vi "ME_acquire_13_DeltaForce_Daq.vi"() -> ()   [LabVIEW 2015]
doc: "Use this template to build a producer/consumer design pattern. Use this template when you need to execute a process, such as data analysis, when a data source, such as a triggered acquisition, produces data at an uneven rate and you need to execute the process when the data becomes available."
uses:
  Mode.ctl
  oxford_driver/Oxford Drivers/BUSGEN.LLB/OxfordAddress.ctl
  <vilib>/Analysis/baseanly.llb/Mean (DBL).vi
  <vilib>/DAQmx/read.llb/DAQmx Read (Analog 1D DBL 1Chan NSamp).vi
  <vilib>/DAQmx/create/channels.llb/DAQmx Create Channel (AI-Voltage-Basic).vi
  <vilib>/DAQmx/configure/timing.llb/DAQmx Timing (Sample Clock).vi
  <vilib>/Utility/file.llb/Write Delimited Spreadsheet (DBL).vi
  <vilib>/DAQmx/miscellaneous.llb/DAQmx Fill In Error Info.vi
  <vilib>/express/express arith-compare/Formula/XNode/ExpressFormulaBlockNode.xnode
  <vilib>/Analysis/NI_AALBase.lvlib
panel:
  out "concatenated string":string
  out "remaining elements 2":T1(array[cluster])
  out "Actual mean":dbl format="%0.6f"
  in  "Averaged dt":dbl[][](array[numeric])
  in  "Averaged P(B)":dbl[][](array[numeric])
  out "LockInR":dbl
  out "deltaUaux":dbl
  out "Actual Voltage (V)":dbl caption="Actual AuxV" step=0.1
  in  "Stop":bool
  out "SaveSweep":bool=TRUE
  out "Measurement File_dn":path
  out "Measurement File_up":path
  out "Measurement File_average":path
  out "Actual Polarization":dbl
  in  "Reset IB?":bool
  in  "First?":bool
  in  "Save Period":dbl=1.0
  out "Averaged I(B)":dbl[][](array[numeric])
  out "P(uC/mm^2)":dbl[](array[numeric])
  in  "Sweep":bool
  out "Offset array":dbl[](array[numeric])
  in  "stop 2":bool
  in  "dB":dbl=0.005
  out "appended array":dbl[][](array[numeric])
  out "Actual B Field (T)":dbl
  out "Actual Temperature (K)":dbl
  out "Actual Current (pA)":dbl
  in  "Tab Control":T2(tab)
  in  "Max temperature (K)":dbl=20.0
  in  "Min Temperature (K)":dbl=4.5
  out "P(T)":cluster{"yi":dbl[], dbl[]}(graph)
  out "I(T)":cluster{dbl[], dbl[]}(graph)
  in  "Set temperature (K)":dbl=4.5
  in  "Temp Ramping Rate (K/min)":dbl=10.0
  in  "Heater Range":enum16{"Off", "Low", "Medium", "High"}(ring)
  in  "Heater On/Off":bool
  out "Setpoint Temperature (K)":dbl
  out "I(B) 3":cluster{dbl[], dbl[]}[](graph)
  out "I(B) /Averaged/":cluster{"B array":dbl[], dbl[]}[](graph)
  out "P(B) /Averaged/":cluster{"B array":dbl[], dbl[]}[](graph)
  out "P(B)":cluster{"yi":dbl[], dbl[]}(graph)
  in  "Set Field (T)":dbl
  in  "Go to Set":bool
  in  "Sweep Rate (T/min)":dbl=2.0 format="%.6f"
  in  "Field To Zero":bool
  out "Target Field":dbl
  in  "Min Field (T)":dbl
  in  "Max Field (T)":dbl=0.15
  in  "Threshold B (T)":dbl
  out "Up/Down":bool
  in  "Max count array":i32[](array[numeric])=[2, 1, 0, 0, 0, 9, 10, 11, 12]
  in  "secs to wait":dbl=180.0
  out "Wait (s)":dbl
  in  "Directory":string
  out "Finished":bool=TRUE
  out "Step Rate":bool
  out "New":bool=TRUE
  in  "Temperature Array":dbl[](array[numeric])=[4.5, 5.0, 6.0, 7.0, 8.0, 9.0, 10.0, 11.0, 12.0]
  in  "Sweep Rate Array":dbl[](array[numeric])=[2.0, 1.0, 0.5, 0.1, 0.05, 9.0, 10.0, 11.0, 12.0]
  in  "Record ALL":bool
  in  "Max Countl":i32
  out "i":i32
  out "j":i32
  out "Step Temp":bool
  in  "FileName":string
  in  "Measure Noise":bool
  in  "Cycles":i32
  in  "maximum value":dbl=10.0 format="%0.2f"
  in  "minimum value":dbl=-10.0 format="%0.2f"
  in  "physical channels":tag="Dev1/ai1"
  out "PSD (pA/Hz^1/2) Peaks Removed":cluster{"f0":dbl, "df":dbl, "magnitude":dbl[]}(graph)
  out "PSD (pA/Hz^1/2)":cluster{"f0":dbl, "df":dbl, "magnitude":dbl[]}(graph)
  out "Current (pA) Filtered":waveform(dbl)(graph)
  out "Current (pA)":dbl[](graph)
  in  "Samples per channel":i32=1000
  in  "Rate":dbl=1000.0 format="%0.2f"
  in  "Cut-Off Frequency":dbl=100.0 caption="Lower Cut-Off"
  in  "Filter On":bool
  in  "Keithley (IV conv) averaging":i32=10
  in  "Lock_in_Amplifier":refnum<visa-resource-name>="GPIB0::5::INSTR"
  out "Dc offset":dbl
  in  "Calibrate":bool
  in  "IV converter":refnum<visa-resource-name>="GPIB0::20::INSTR"
  in  "Magnetic Field":refnum<visa-resource-name>="GPIB0::21::INSTR"
  out "Time Lag":dbl=0.0500025749206543
  in  "Lake Shore":refnum<visa-resource-name>="GPIB0::11::INSTR"
  in  "Temp Refresh (s)":dbl=0.1
  in  "Sampling rate (Hz)":dbl=10.0
  in  "Gain (V/A)":dbl=1000000000.0
  in  "Sample area (mm^2)":dbl=1.0
  out "B_V":cluster{dbl[], "Best Linear Fit":dbl[]}[](graph)=[{[-0.00769241141, -0.00768011662, -0.0029394633, 0.00271952438, 0.00937200583, 0.0154641889, 0.0217080684, 0.0281692221, 0.0344763397, 0.0407091529, 0.0473661569, 0.0541476438, 0.0611164384, 0.0676637725, 0.073937413, 0.0801511723, 0.0863882257, 0.0933787866, 0.0997676928, 0.106163316, 0.113953626, 0.118979018, 0.126030157, 0.132855724, 0.13883398, 0.14631074, 0.153030676, 0.159156864, 0.165801088, 0.17248087, 0.178555009, 0.185285367, 0.192834407, 0.198751051, 0.205413053, 0.212847389, 0.219477697, 0.225574642, 0.232225854, 0.239015189, 0.245675966, 0.252411162, 0.258453848, 0.265211852, 0.271251534, 0.277801221, 0.284008329, 0.291402813, 0.297970768, 0.304082546, 0.310761405, 0.317366634, 0.323522001, 0.330123184, 0.336841279, 0.343557963, 0.349608435, 0.356238003, 0.363590921, 0.370338319, 0.376962983], "Best Linear Fit"=[0.0, 0.0015, 0.0035, 0.0056, 0.0076, 0.0096, 0.0116, 0.0136, 0.0156, 0.0177, 0.0197, 0.0219, 0.0239, 0.0259, 0.0279, 0.0299, 0.032, 0.034, 0.036, 0.038, 0.04, 0.042, 0.0441, 0.046, 0.048, 0.05, 0.052, 0.054, 0.056, 0.058, 0.06, 0.0621, 0.0643, 0.0663, 0.0684, 0.0704, 0.0725, 0.0745, 0.0765, 0.0787, 0.0807, 0.0827, 0.0847, 0.0868, 0.0888, 0.0908, 0.0928, 0.0948, 0.0968, 0.0988, 0.1008, 0.1028, 0.1048, 0.1069, 0.1091, 0.1111, 0.1131, 0.1152, 0.1173, 0.1193, 0.1213]}, {[-0.00769241141, -0.00768011662, -0.0029394633, 0.00271952438, 0.00937200583, 0.0154641889, 0.0217080684, 0.0281692221, 0.0344763397, 0.0407091529, 0.0473661569, 0.0541476438, 0.0611164384, 0.0676637725, 0.073937413, 0.0801511723, 0.0863882257, 0.0933787866, 0.0997676928, 0.106163316, 0.113953626, 0.118979018, 0.126030157, 0.132855724, 0.13883398, 0.14631074, 0.153030676, 0.159156864, 0.165801088, 0.17248087, 0.178555009, 0.185285367, 0.192834407, 0.198751051, 0.205413053, 0.212847389, 0.219477697, 0.225574642, 0.232225854, 0.239015189, 0.245675966, 0.252411162, 0.258453848, 0.265211852, 0.271251534, 0.277801221, 0.284008329, 0.291402813, 0.297970768, 0.304082546, 0.310761405, 0.317366634, 0.323522001, 0.330123184, 0.336841279, 0.343557963, 0.349608435, 0.356238003, 0.363590921, 0.370338319, 0.376962983], "Best Linear Fit"=[0.002353460844818253, 0.002357267374965663, 0.003824997997530172, 0.005577049655813272, 0.007636692089275871, 0.009522863265806463, 0.01145600043639222, 0.013456406815525209, 0.015409122826751182, 0.01733883381400479, 0.019399876452181594, 0.021499459635718428, 0.023657034245452215, 0.025684122519169482, 0.027626473848249778, 0.02955028565017564, 0.03148130942513291, 0.03364562299316916, 0.03562366117513693, 0.037603778974812686, 0.040015698972850115, 0.04157158615356273, 0.04375465501257369, 0.04586788562152819, 0.0477187843918964, 0.050033627699098075, 0.05211415440778254, 0.05401085368533849, 0.056067939569859164, 0.05813603439385595, 0.06001661903361471, 0.06210037244704129, 0.06443759401357516, 0.0662694173922171, 0.06833200743687069, 0.07063371605572277, 0.07268649347515121, 0.0745741389696738, 0.07663338837489471, 0.07873540137051047, 0.08079761214887074, 0.08288286343195213, 0.08475371006132383, 0.08684602281837933, 0.08871593939391825, 0.09074375613756333, 0.09266550866283872, 0.09495487889775463, 0.09698835150804998, 0.09888058937557581, 0.10094839843403076, 0.10299341126621803, 0.10489914451207855, 0.10694290468187984, 0.10902286140750632, 0.11110238128028392, 0.11297563849525552, 0.11502818680688229, 0.1173046879946565, 0.11939371707962458, 0.12144474708765744]}]
  out "V_I":cluster{dbl[], "Best Linear Fit":dbl[]}[](graph)=[{[0.0, 0.012, 0.026, 0.04, 0.054, 0.068, 0.081, 0.096, 0.11, 0.124, 0.138, 0.153, 0.167, 0.18, 0.195, 0.208, 0.223, 0.236, 0.251, 0.265, 0.279, 0.292, 0.306, 0.32, 0.334, 0.348, 0.362, 0.375, 0.389, 0.403, 0.417, 0.432, 0.446, 0.46, 0.475, 0.489, 0.504, 0.517, 0.531, 0.546, 0.56, 0.574, 0.588, 0.602, 0.616, 0.63, 0.644, 0.658, 0.672, 0.685, 0.699, 0.713, 0.727, 0.742, 0.755, 0.77, 0.784, 0.799, 0.814, 0.827, 0.841], "Best Linear Fit"=[-0.00769241141, -0.00768011662, -0.0029394633, 0.00271952438, 0.00937200583, 0.0154641889, 0.0217080684, 0.0281692221, 0.0344763397, 0.0407091529, 0.0473661569, 0.0541476438, 0.0611164384, 0.0676637725, 0.073937413, 0.0801511723, 0.0863882257, 0.0933787866, 0.0997676928, 0.106163316, 0.113953626, 0.118979018, 0.126030157, 0.132855724, 0.13883398, 0.14631074, 0.153030676, 0.159156864, 0.165801088, 0.17248087, 0.178555009, 0.185285367, 0.192834407, 0.198751051, 0.205413053, 0.212847389, 0.219477697, 0.225574642, 0.232225854, 0.239015189, 0.245675966, 0.252411162, 0.258453848, 0.265211852, 0.271251534, 0.277801221, 0.284008329, 0.291402813, 0.297970768, 0.304082546, 0.310761405, 0.317366634, 0.323522001, 0.330123184, 0.336841279, 0.343557963, 0.349608435, 0.356238003, 0.363590921, 0.370338319, 0.376962983]}, {[0.0, 0.012, 0.026, 0.04, 0.054, 0.068, 0.081, 0.096, 0.11, 0.124, 0.138, 0.153, 0.167, 0.18, 0.195, 0.208, 0.223, 0.236, 0.251, 0.265, 0.279, 0.292, 0.306, 0.32, 0.334, 0.348, 0.362, 0.375, 0.389, 0.403, 0.417, 0.432, 0.446, 0.46, 0.475, 0.489, 0.504, 0.517, 0.531, 0.546, 0.56, 0.574, 0.588, 0.602, 0.616, 0.63, 0.644, 0.658, 0.672, 0.685, 0.699, 0.713, 0.727, 0.742, 0.755, 0.77, 0.784, 0.799, 0.814, 0.827, 0.841], "Best Linear Fit"=[-0.015941127780698654, -0.010342478990544012, -0.0038107220686969304, 0.0027210348531501527, 0.009252791774997235, 0.01578454869684432, 0.02184975155284518, 0.028848062540538483, 0.03537981946238557, 0.041911576384232645, 0.048443333306079736, 0.05544164429377303, 0.061973401215620116, 0.06803860407162098, 0.07503691505931429, 0.08110211791531513, 0.08810042890300844, 0.0941656317590093, 0.10116394274670261, 0.1076956996685497, 0.11422745659039678, 0.12029265944639762, 0.1268244163682447, 0.1333561732900918, 0.13988793021193888, 0.14641968713378595, 0.15295144405563305, 0.15901664691163392, 0.165548403833481, 0.1720801607553281, 0.17861191767717516, 0.18561022866486845, 0.19214198558671555, 0.19867374250856262, 0.20567205349625592, 0.212203810418103, 0.2192021214057963, 0.22526732426179719, 0.23179908118364426, 0.23879739217133758, 0.24532914909318465, 0.2518609060150317, 0.2583926629368788, 0.2649244198587259, 0.271456176780573, 0.27798793370242003, 0.28451969062426713, 0.29105144754611423, 0.2975832044679613, 0.3036484073239622, 0.31018016424580924, 0.3167119211676563, 0.3232436780895034, 0.3302419890771967, 0.3363071919331976, 0.3433055029208909, 0.34983725984273795, 0.35683557083043127, 0.36383388181812454, 0.3698990846741254, 0.3764308415959725]}]
  out "B0 (T)":dbl=0.0026443907573365636
  out "B/V (T/V)":dbl=0.3027997253900218
  out "I0 (A)":dbl=-0.008736391445912099
  out "V/I (Ohm)":dbl=0.4773805959957447
  in  "Offset?":bool
  in  "Magnet":bool=TRUE
  in  "Ramp":bool=TRUE
  in  "DaQ":bool
  in  "Moving average":i8=10
  in  "Sample Rate":dbl=1000.0
  in  "Number of Samples":i32=100
  in  "Physical Channel":tag="kartya/ai0"
  in  "Min Voltage":dbl=-5.0
  in  "Max Voltage":dbl=5.0
  in  "Terminal Configuration":i32(ring)=-1 items=["default"=-1, "RSE"=10083, "NRSE"=10078, "Differential"=10106, "Pseudodifferential"=12529]
  out "Confirm":bool
  in  "Dwell Time (ms)":u32=1000
  in  "Temp/Magnetic Field":bool
  out "index":i8
  out "Read?":bool
  out "Magnetic Field (T)":dbl[](array[numeric])
  out "Reset":bool
  out "Measured Current (pA)":dbl[](array[numeric])
  out "Elapsed Time (s)":dbl[](array[numeric])
  out "Start time":timestamp
  in  "Enum":T3=enum."Process"
  out "B array":dbl[](array[numeric])
  in  "dB (T)":dbl=0.0025
  in  "Counter":i8
  out "L magnet (H)":dbl
  out "R magnet (mOhm)":dbl
  out "Actual Current (R0)":dbl
  out "Actual Field (T)":dbl
  out "Temperature array":dbl[](array[numeric])
  in  "New Measurement File":bool
  out "Measurement File":path
  out "refnum out":refnum<file>
  in  "Measuring":bool
  in  "Measure /Pause":bool
  in  "stop":bool
  # "DeltaForce"
  # "Discrete"
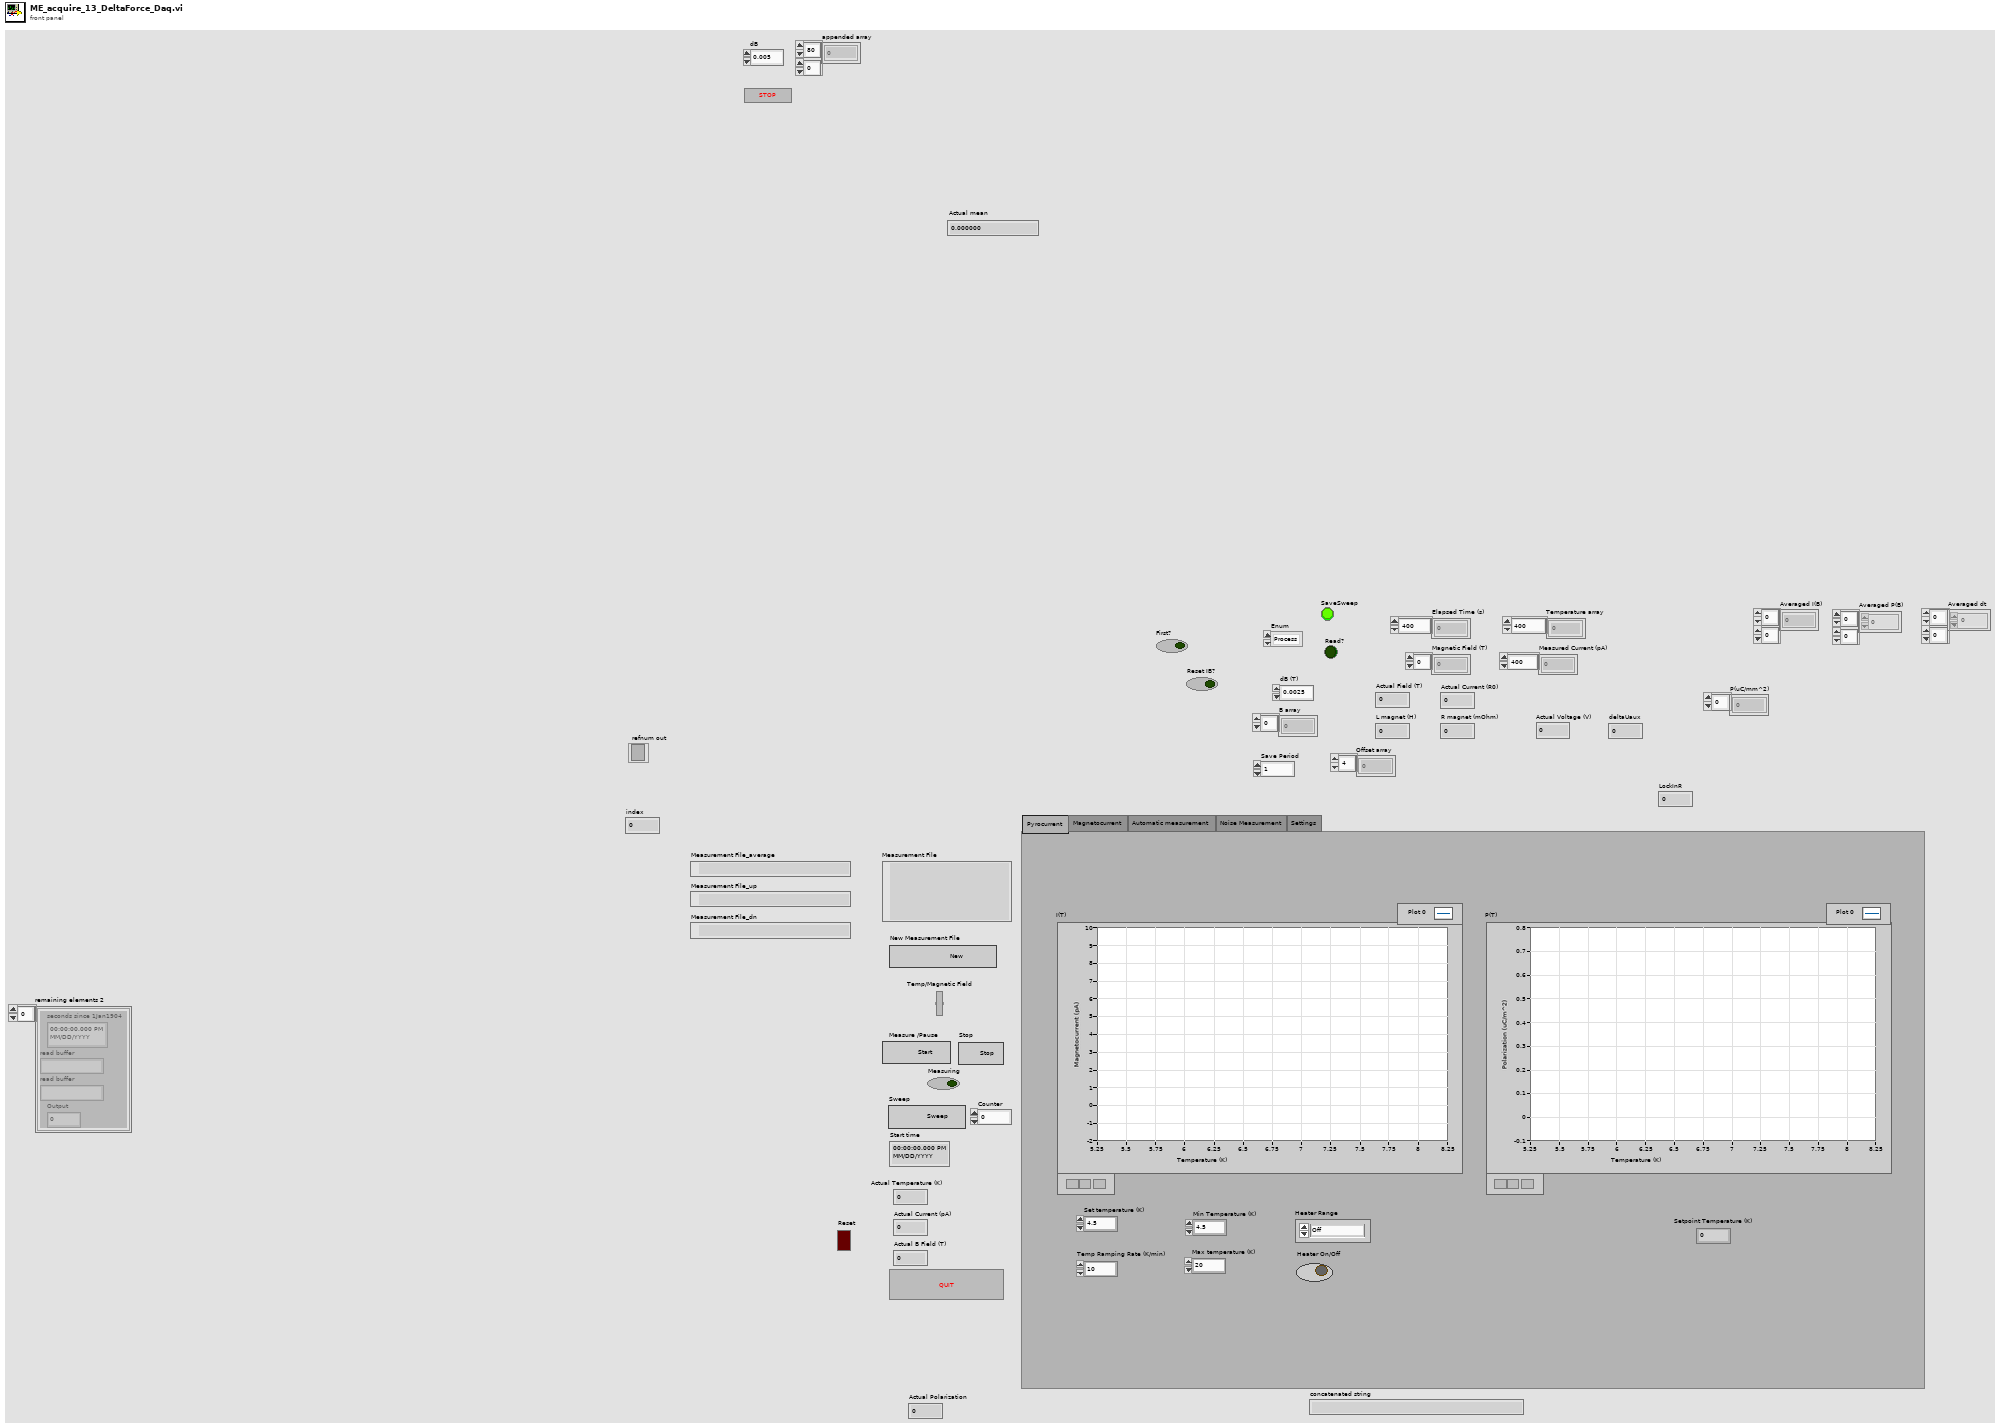
[diagram p1: front panel]
types:
  T1 = cluster{"seconds since 1Jan1904":timestamp, "read buffer":string, "read buffer":string, "Output":dbl}[]
  T2 = enum32{"Pyrocurrent", "Magnetocurrent", "Automatic measurement", "Noise Measurement", "Settings"}
  T3 = typedef "Mode.ctl" = enum16{"Offset", "Process", "Sweep", "StepOxford", "StepDelta", "Plot", "Save", "New", "Return", ""}
  T4 = cluster{"seconds since 1Jan1904":timestamp, "read buffer":string, "read buffer":string, "Output":dbl}
  T5 = enum16{"open", "replace", "create", "open or create", "replace or create", "replace or create with confirmation"}
  T6 = typedef "OxfordAddress.ctl" = cluster{"Com Port":i32, "ISOBUS Address":i32, "GPIB Address":i16, "Communication":enum16{"RS232", "ISOBUS", "GPIB", "Gateway"}}
  T7 = cluster{"B array":dbl[], "Averaged P(B) Out":dbl[]}
  T8 = cluster{"B array":dbl[], "BaselineSubtracted I(B)":dbl[]}
  T9 = cluster{"B array":dbl[], "Averaged P(B) Out":dbl[]}[]
  T10 = cluster{"B array":dbl[], "BaselineSubtracted I(B)":dbl[]}[]
  T11 = cluster{"I array out (A)":dbl[], "V array out (V)":dbl[]}
  T12 = cluster{"I array out (A)":dbl[], "Best Linear Fit":dbl[]}
  T13 = cluster{"V array out (V)":dbl[], "B array Out":dbl[]}
  T14 = cluster{"V array out (V)":dbl[], "Best Linear Fit 2":dbl[]}
  T15 = cluster{"I array out (A)":dbl[], "Best Linear Fit":dbl[]}[]
  T16 = cluster{"V array out (V)":dbl[], "Best Linear Fit 2":dbl[]}[]
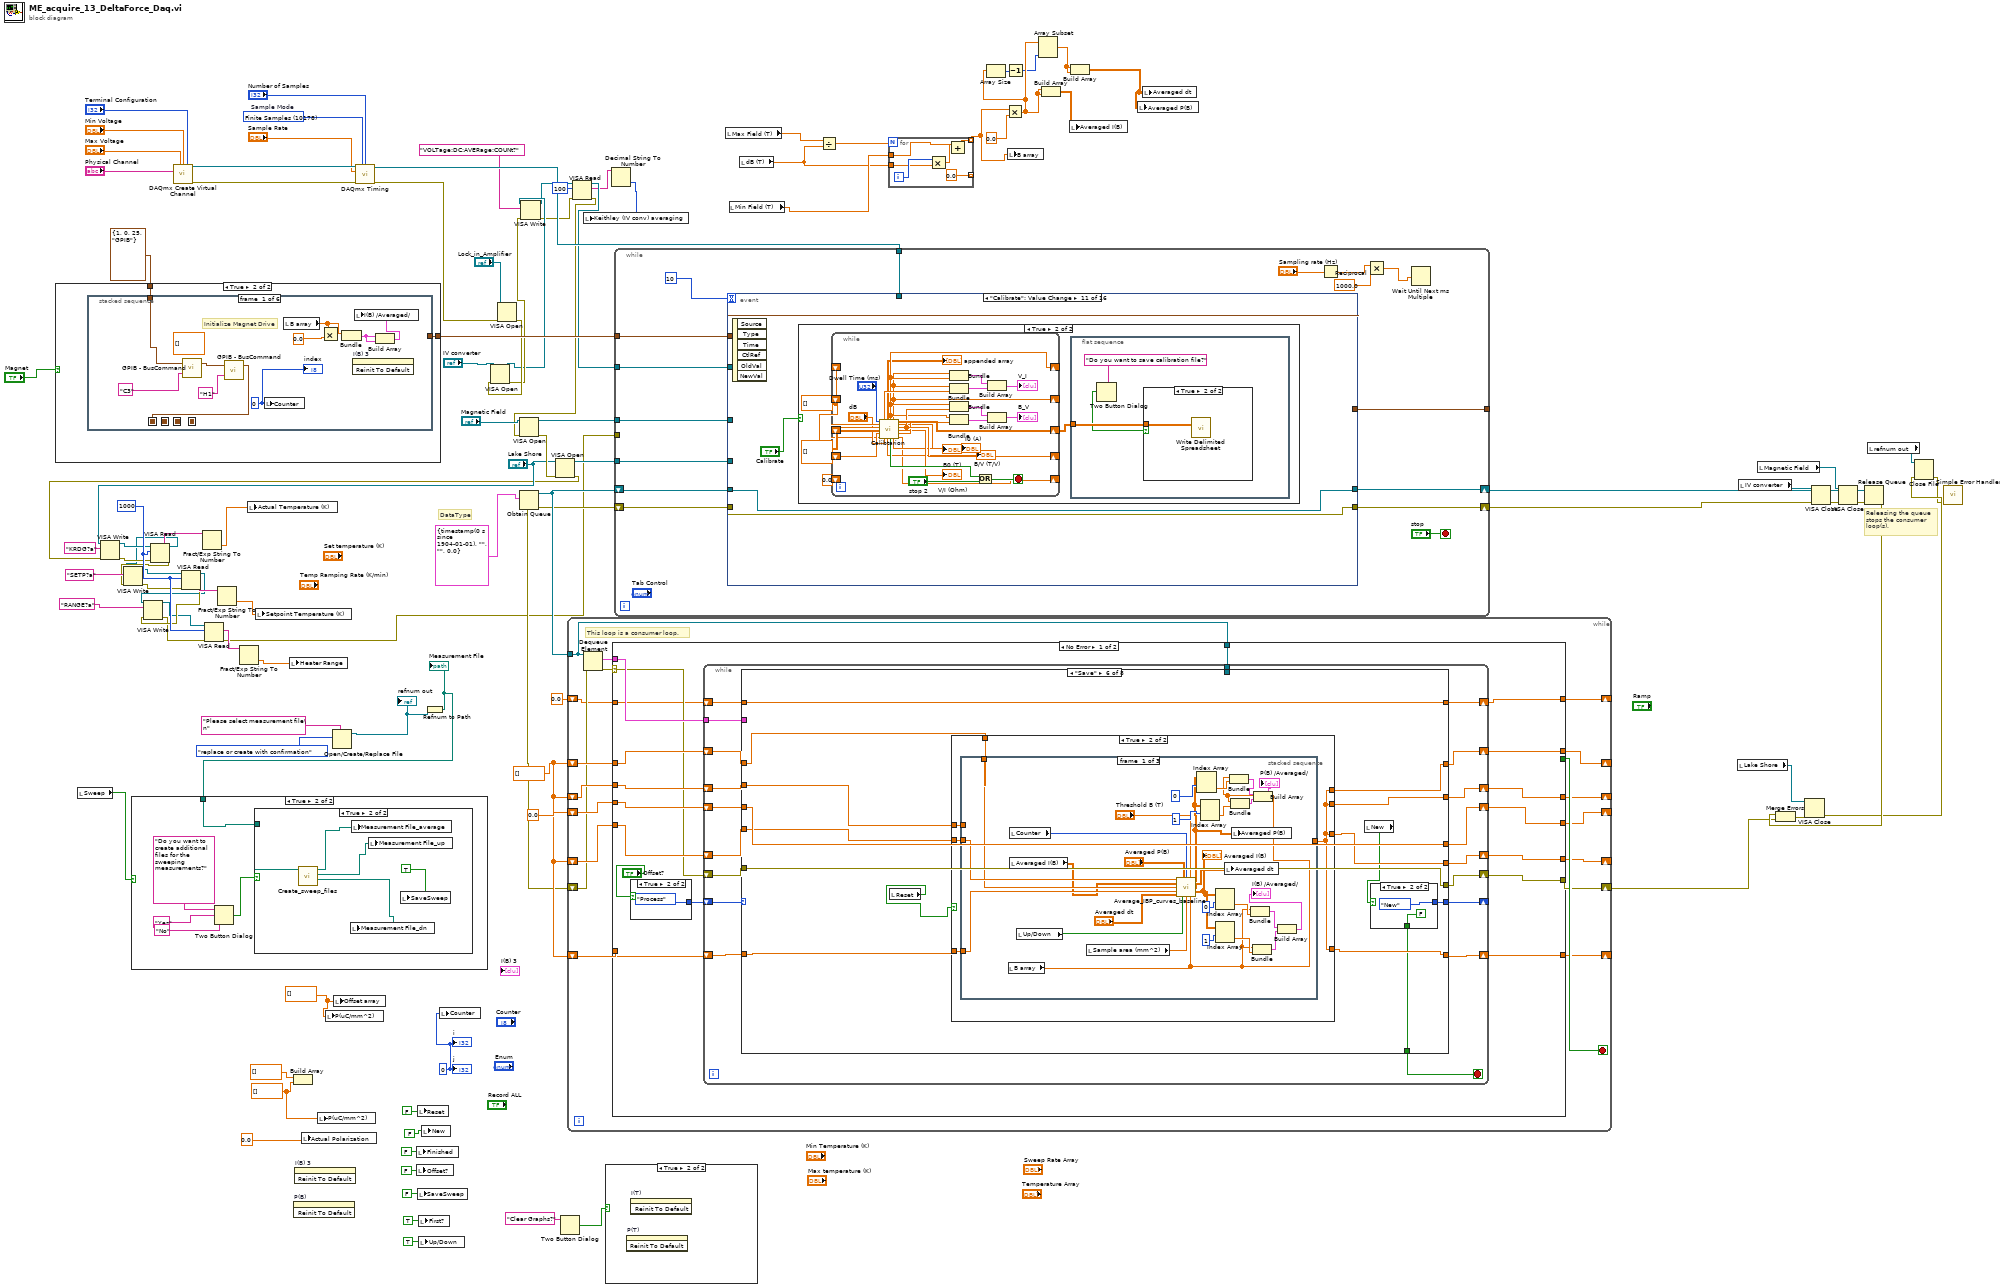
[diagram p0: block diagram]
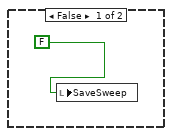
[diagram p4: hidden frame]
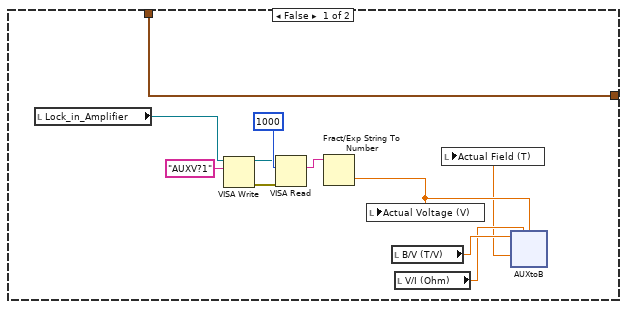
[diagram p5: hidden frame]
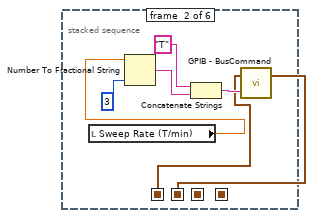
[diagram p6: hidden frame]
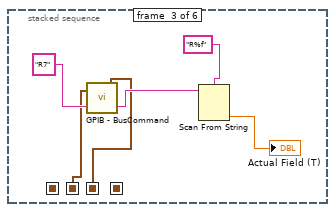
[diagram p7: hidden frame]
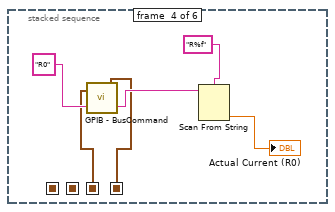
[diagram p8: hidden frame]
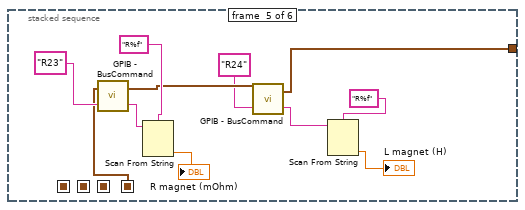
[diagram p9: hidden frame]
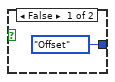
[diagram p11: hidden frame]
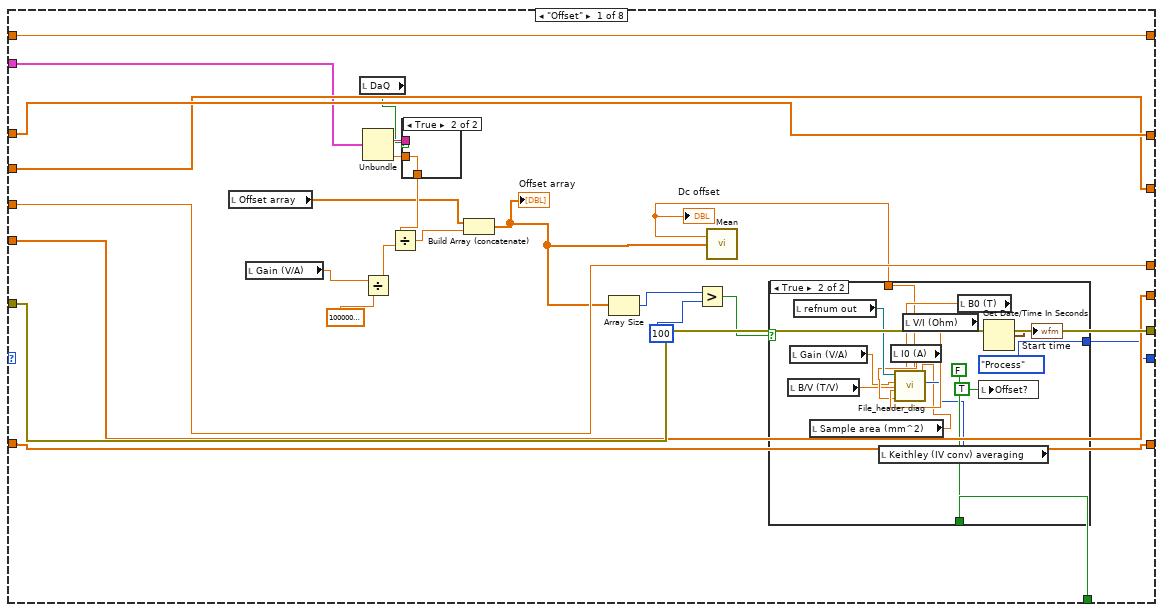
[diagram p12: hidden frame]
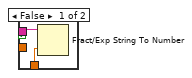
[diagram p13: hidden frame]
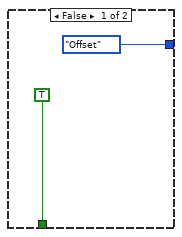
[diagram p14: hidden frame]
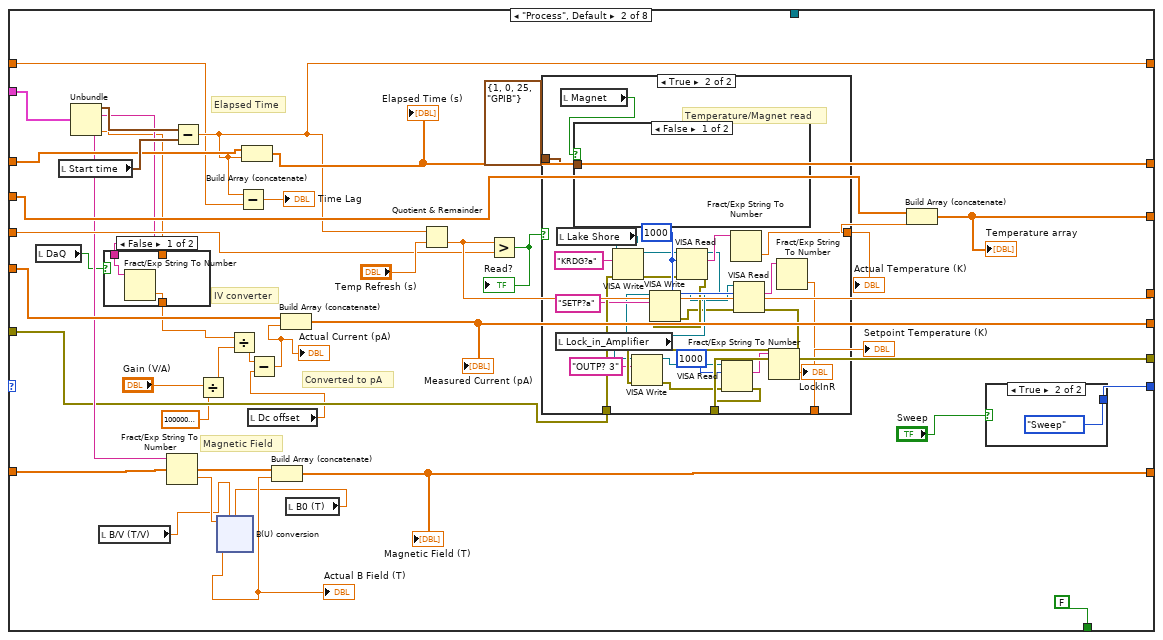
[diagram p15: hidden frame]
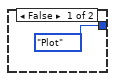
[diagram p17: hidden frame]
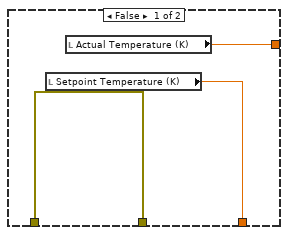
[diagram p18: hidden frame]
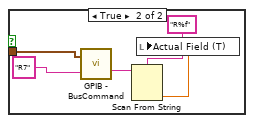
[diagram p19: hidden frame]
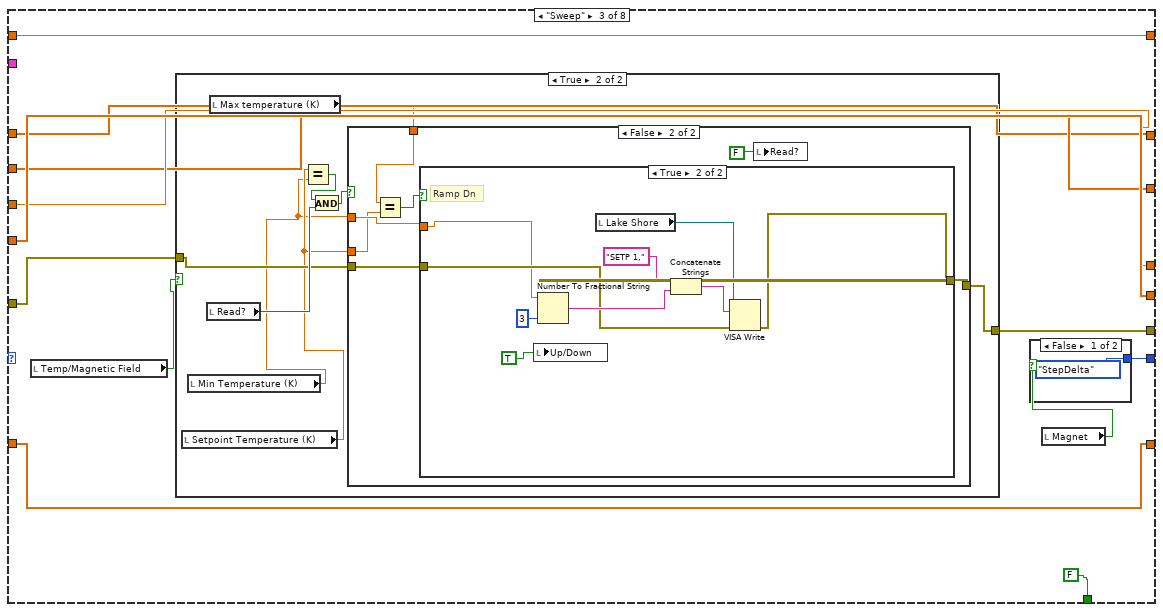
[diagram p20: hidden frame]
diagram:
  w22 = 10178 items=["Finite Samples"=10178, "Continuous Samples"=10123, "Hardware Timed Single Point"=12522]  # Sample Mode
  w49 = u32 1000 ("byte count")
  w60 = 0 ("j")
  w57 = dbl[] []
  w75 = dbl[] []
  w81 = dbl[] []
  # "DataType"
  # "Releasing the queue stops the consumer loop(s)."
  n1 = case shown="True" "Magnet" {
    tunnel: T6 {"Com Port"=1, "ISOBUS Address"=0, "GPIB Address"=25, "Communication"=enum."GPIB"} ("Address") -> [w115 w129]
    tunnel: [w115 w128] -> w87
    frame False {
      n2 = local read "Lock_in_Amplifier"() -> (w109:refnum<visa-resource-name>)
      n3 = VISA Write(VISA resource name=w109, write buffer="AUXV?1") -> (VISA resource name out=w110:refnum<visa-resource-name>, error out=w114:errorcluster)  [unwired: 1 in, 1 out]
      n4 = VISA Read(VISA resource name=w110, byte count=u32 1000, error in (no error)=w114) -> (read buffer=w113:string)  [unwired: 3 out]
      n5 = Fract/Exp String To Number(string=w113) -> (number=w106:dbl)  [unwired: 3 in, 1 out]
      n6 = local write "Actual Voltage (V)"(w106) -> ()
      n7 = local read "B/V (T/V)"() -> (w108:dbl)
      n8 = local read "V/I (Ohm)"() -> (w107:dbl)
      n9 = xnode "AUXtoB"("BpV"=w108, "Rm"=w107, "Aux"=w106) -> ("Result"=w105:dbl)  [unwired: 1 in, 1 out]
      n10 = local write "Actual Field (T)"(w105) -> ()
    }
    frame True {
      n11 = stacked-sequence {
        seq-local: [w137 _ _ _ _ _] -> [_ w142 _ _ _ _]
        seq-local: [_ w141 _ _ _ _] -> [_ _ w149 _ _ _]
        seq-local: [_ _ w148 _ _ _] -> [_ _ _ w155 _ _]
        seq-local: [_ _ _ w154 _ _] -> [_ _ _ _ w166 _]
        tunnel: w129 -> [w139 _ _ _ _ _]
        tunnel: [_ _ _ _ w164 _] -> w128
        frame #0 {
          (unwired) dbl[][] []
          w135 = i8 0 ("Counter")
          # "Initialize Magnet Drive"
          n12 = call "GPIB - BusCommand.vi"("Command"="C3", "Address"=w139) -> ("Address(thru)"=w138:T6)  [unwired: 1 out]
          n13 = call "GPIB - BusCommand.vi"("Command"="H1", "Address"=w138) -> ("Address(thru)"=w137:T6)  [unwired: 1 out]
          n14 = local write "Counter"(w135) -> ()
          n15 = local read "B array"() -> (w133:dbl[])
          n16 = Multiply(x=w133, y=0.0) -> (x*y=w132:dbl[])
          n17 = Bundle("B array"=w133, w132) -> (w131:cluster{"B array":dbl[], dbl[]})  [unwired: 1 in]
          n18 = invoke on="I(B) 3" class="XYGraph (strict)" method="Reinit To Default"() -> ()  [unwired: 3 in, 3 out]
          n19 = Build Array(w131, w131) -> (w130:cluster{"B array":dbl[], dbl[]}[])
          n20 = local write "I(B) /Averaged/"(w130) -> ()
          "index" <- w135
        }
        frame #1 {
          n21 = local read "Sweep Rate (T/min)"() -> (w143:dbl)
          n22 = Number To Fractional String(number=w143, precision (6)=i16 3) -> (F-format string=w145:string)  [unwired: 2 in]
          n23 = Concatenate Strings("T" ("format string"), w145) -> (w144:string)
          n24 = call "GPIB - BusCommand.vi"("Command"=w144, "Address"=w142) -> ("Address(thru)"=w141:T6)  [unwired: 1 out]
        }
        frame #2 {
          n25 = call "GPIB - BusCommand.vi"("Command"="R7" ("format string"), "Address"=w149) -> ("Reply"=w153:string, "Address(thru)"=w148:T6)
          n26 = Scan From String(format string="R%f" ("remaining string"), input string=w153) -> (output 1=→"Actual Field (T)":dbl)  [unwired: 3 in, 3 out]
        }
        frame #3 {
          n27 = call "GPIB - BusCommand.vi"("Command"="R0" ("format string"), "Address"=w155) -> ("Reply"=w159:string, "Address(thru)"=w154:T6)
          n28 = Scan From String(format string="R%f" ("remaining string"), input string=w159) -> (output 1=→"Actual Current (R0)":dbl)  [unwired: 3 in, 3 out]
        }
        frame #4 {
          n29 = call "GPIB - BusCommand.vi"("Command"="R23" ("format string"), "Address"=w166) -> ("Reply"=w170:string, "Address(thru)"=w165:T6)
          n30 = Scan From String(format string="R%f" ("remaining string"), input string=w170) -> (output 1=→"R magnet (mOhm)":dbl)  [unwired: 3 in, 3 out]
          n31 = call "GPIB - BusCommand.vi"("Command"="R24" ("format string"), "Address"=w165) -> ("Reply"=w162:string, "Address(thru)"=w164:T6)
          n32 = Scan From String(format string="R%f" ("remaining string"), input string=w162) -> (output 1=→"L magnet (H)":dbl)  [unwired: 3 in, 3 out]
        }
        frame #5 {
        }
      }
    }
  }
  n33 = local read "Sweep"() -> (w65:bool)
  n34 = call-poly <vilib>:"DAQmx Create Virtual Channel.vi"("maximum value"="Max Voltage", "minimum value"="Min Voltage", "input terminal configuration"="Terminal Configuration", "physical channels"="Physical Channel") -> ("task out"=w20:refnum<k21>, "error out"=w21:errorcluster)  [unwired: 10 in]
  n35 = Build Array(dbl[] [], w57) -> ()  [unwired: 1 out]
  n36 = invoke on="P(B)" class="XYGraph (strict)" method="Reinit To Default"() -> ()  [unwired: 3 in, 3 out]
  n37 = invoke on="I(B) 3" class="XYGraph (strict)" method="Reinit To Default"() -> ()  [unwired: 3 in, 3 out]
  n38 = local write "Actual Polarization"(0.0 ("Actual Polarization")) -> ()
  n39 = local write "P(uC/mm^2)"(w57) -> ()
  n40 = local write "P(uC/mm^2)"(w75) -> ()
  n41 = Open/Create/Replace File(prompt="Please select measurement file\n", operation (0:open)=T5."replace or create with confirmation") -> (refnum out=w84:refnum<file>)  [unwired: 4 in, 2 out]
  "refnum out" <- w84
  n42 = local write "Offset array"(w75) -> ()
  n43 = call-poly <vilib>:"DAQmx Timing.vi"("task/channels in"=w20, "sample mode"=w22, "samples per channel"="Number of Samples", "rate"="Sample Rate", "error in"=w21) -> ("task out"=w12:refnum<k21>, "error out"=w13:errorcluster)  [unwired: 9 in]
  n44 = local write "Finished"(FALSE ("Finished")) -> ()
  n45 = local write "Offset?"(FALSE ("Offset?")) -> ()
  n46 = local write "Reset"(FALSE ("Reset")) -> ()
  n47 = local write "SaveSweep"(FALSE ("SaveSweep")) -> ()
  n48 = local write "First?"(TRUE ("First?")) -> ()
  n49 = local write "Up/Down"(TRUE ("Up/Down")) -> ()
  n50 = local write "New"(FALSE ("New")) -> ()
  n51 = Refnum to Path(1:w84) -> (0:w64:path)
  "Measurement File" <- w64
  n52 = case shown="True" w65 {
    tunnel: w64 -> [_ w171]
    frame False {
    }
    frame True {
      n53 = Two Button Dialog(message="Do you want to create additional files for the sweeping measurements?" ("string"), 1:"No" ("F button name (\"Cancel\")"), 2:"Yes" ("T button name (\"OK\")")) -> (T button?=w173:bool)
      n54 = case shown="True" w173 {
        tunnel: w171 -> [_ w181]
        frame False {
          n55 = local write "SaveSweep"(FALSE ("SaveSweep")) -> ()
        }
        frame True {
          n56 = call "Create_sweep_files.vi"("Measurement File"=w181) -> ("Path 3"=w178:path, "Path 2"=w179:path, "Path"=w180:path)  [unwired: 8 in]
          n57 = local write "Measurement File_dn"(w178) -> ()
          n58 = local write "Measurement File_average"(w180) -> ()
          n59 = local write "Measurement File_up"(w179) -> ()
          n60 = local write "SaveSweep"(TRUE) -> ()
        }
      }
    }
  }
  n61 = local write "Counter"(w60) -> ()
  n62 = VISA Open(error in (no error)=w13, VISA resource name="Lock_in_Amplifier") -> (error out=w32:errorcluster)  [unwired: 3 in, 1 out]
  n63 = VISA Open(error in (no error)=w32, VISA resource name="IV converter") -> (VISA resource name=w9:refnum<visa-resource-name>, error out=w10:errorcluster)  [unwired: 3 in]
  n64 = Obtain Queue(element data type=T4 {"seconds since 1Jan1904"=timestamp(0 s since 1904-01-01), "read buffer"="", "read buffer"="", "Output"=0.0} ("output cluster")) -> (queue out=w104:refnum<queue>, error out=w79:errorcluster)  [unwired: 4 in, 1 out]
  n65 = VISA Write(VISA resource name=w9, write buffer="VOLTage:DC:AVERage:COUNt?", error in (no error)=w10) -> (VISA resource name out=w5:refnum<visa-resource-name>, error out=w7:errorcluster)  [unwired: 1 out]
  n66 = Two Button Dialog(message="Clear Graphs?") -> (T button?=w59:bool)  [unwired: 2 in]
  n67 = while {
    tunnel: w104 -> [w182]
    shift-right: [w195] -> _
    shift-left: w81 -> [w194]
    shift-right: [w193] -> _
    shift-left: w81 -> [w192]
    shift-right: [w191] -> _
    shift-left: w81 -> [w190]
    shift-right: [w189] -> _
    shift-left: 0.0 -> [w188]
    shift-right: [w187] -> _
    shift-left: w81 -> [w186]
    shift-right: [w196] -> w92
    shift-left: w79 -> [w185]
    shift-right: [w184] -> _
    shift-left: 0.0 -> [w183]
    stop <- w197 stop-if-true
    # "This loop is a consumer loop."
    n68 = Dequeue Element(queue=w182, error in (no error)=w185) -> (element=w198:T4, error out=w199:errorcluster)  [unwired: 1 in, 2 out]
    n69 = case shown="No Error" w199 {
      selector: w199 -> [w205 w881]
      tunnel: w198 -> [w216 _]
      tunnel: [_ TRUE] -> w197
      tunnel: [w204 w881] -> w196
      tunnel: [w215 w880] -> w195
      tunnel: w194 -> [w214 w880]
      tunnel: [w213 w877] -> w193
      tunnel: w192 -> [w212 w877]
      tunnel: [w211 w876] -> w191
      tunnel: w190 -> [w210 w876]
      tunnel: [w209 w878] -> w189
      tunnel: w188 -> [w208 w878]
      tunnel: [w207 w879] -> w187
      tunnel: w186 -> [w206 w879]
      tunnel: [w203 w875] -> w184
      tunnel: w183 -> [w202 w875]
      tunnel: w182 -> [w200 _]
      frame No Error {
        n70 = case shown="True" "Offset?" {
          tunnel: [Mode."Offset" ("Enum") Mode."Process" ("Enum")] -> w217
          frame False {
          }
          frame True {
          }
        }
        n71 = while {
          shift-right: [w226] -> _
          shift-left: w217 -> [w238]
          tunnel: w216 -> [w237]
          shift-right: [w236] -> w215
          shift-left: w214 -> [w235]
          shift-right: [w228] -> w207
          shift-left: w206 -> [w227]
          shift-right: [w230] -> w209
          shift-left: w208 -> [w229]
          shift-right: [w234] -> w213
          shift-left: w212 -> [w233]
          shift-right: [w224] -> w204
          shift-left: w205 -> [w225]
          shift-right: [w232] -> w211
          shift-left: w210 -> [w231]
          shift-right: [w222] -> w203
          shift-left: w202 -> [w221]
          tunnel: w200 -> [w220]
          stop <- w223 stop-if-true
          n72 = case shown="\"Save\"" w238 {
            selector: w238 -> [_ _ _ _ _ _ _ w868]
            tunnel: w237 -> [w256 w319 _ _ _ _ _ _]
            tunnel: [w262 w316 w377 w492 w554 w627 w709 w873] -> w236
            tunnel: w235 -> [w262 w309 w377 w492 w554 w623 w709 w873]
            tunnel: [w257 w315 w380 w489 w556 w629 w707 w870] -> w234
            tunnel: w233 -> [w257 w314 w380 w489 w556 w624 w707 w870]
            tunnel: [w258 w313 w382 w487 w551 w630 w705 w867] -> w232
            tunnel: w231 -> [w258 w312 w382 w487 w551 w625 w705 w867]
            tunnel: [w260 w308 w379 w490 w552 w633 0.0 w871] -> w230
            tunnel: w229 -> [w260 w307 w379 w490 w552 w633 _ w871]
            tunnel: [w261 w304 w378 w491 w553 w628 w708 w872] -> w228
            tunnel: w227 -> [w261 w305 w378 w491 w553 w626 w708 w872]
            tunnel: [w245 w302 w375 Mode."Plot" ("Enum") Mode."Save" ("Enum") w634 Mode."Return" ("Enum") w868] -> w226
            tunnel: w225 -> [w259 w300 w384 w484 w559 w632 w701 w869]
            tunnel: [w259 w299 w383 w483 w559 w632 w700 w869] -> w224
            tunnel: [w241 FALSE FALSE FALSE FALSE w621 TRUE TRUE] -> w223
            tunnel: [w244 w296 w376 w485 w555 w631 0.0 w874] -> w222
            tunnel: w221 -> [w244 w295 w376 w485 w555 w631 _ w874]
            tunnel: w220 -> [_ _ _ _ _ _ w699 _]
            frame "Offset" {
              n73 = local read "Offset array"() -> (w250:dbl[])
              n74 = local read "Gain (V/A)"() -> (w254:dbl)
              n75 = local read "DaQ"() -> (w240:bool)
              n76 = Unbundle(w256) -> ("read buffer"=w243:string, "Output"=w239:dbl)  [unwired: 2 out]
              n77 = Divide(x=w254, y=1000000000000.0) -> (x/y=w252:dbl)
              n78 = case shown="True" w240 {
                tunnel: [w264 w265] -> w255
                tunnel: w243 -> [w263 _]
                tunnel: w239 -> [_ w265]
                frame False {
                  n79 = Fract/Exp String To Number(string=w263) -> (number=w264:dbl)  [unwired: 3 in, 1 out]
                }
                frame True {
                }
              }
              n80 = Divide(x=w255, y=w252) -> (x/y=w251:dbl)
              n81 = Build Array (concatenate)(w250, w251) -> (w246:dbl[])
              "Offset array" <- w246
              n82 = Array Size(array=w246) -> (size(s)=w249:i32)
              n83 = Greater?(x=w249, y=100) -> (0:w247:bool)
              n84 = call-poly <vilib>:"Mean.vi"("X"=w246) -> ("mean"=w242:dbl)  [unwired: 1 out]
              "Dc offset" <- w242
              n85 = case shown="True" w247 {
                tunnel: [Mode."Offset" ("Enum") Mode."Process" ("Enum")] -> w245
                tunnel: w242 -> [_ w272]
                tunnel: [TRUE FALSE] -> w241
                frame False {
                }
                frame True {
                  n86 = local read "B/V (T/V)"() -> (w273:dbl)
                  n87 = local read "Gain (V/A)"() -> (w274:dbl)
                  n88 = local read "refnum out"() -> (w278:refnum<file>)
                  n89 = local read "Sample area (mm^2)"() -> (w268:dbl)
                  n90 = local read "Keithley (IV conv) averaging"() -> (w269:i32)
                  n91 = local read "I0 (A)"() -> (w276:dbl)
                  n92 = local read "V/I (Ohm)"() -> (w277:dbl)
                  n93 = local read "B0 (T)"() -> (w275:dbl)
                  n94 = call "File_header_diag.vi"("Averaging"=w269, "Sample area"=w268, "OFFSET"=w272, "B0"=w275, "B/V"=w273, "I0"=w276, "V/I"=w277, "Gain"=w274, "Byte Stream File in"=w278) -> ()  [unwired: 3 in]
                  n95 = local write "Offset?"(TRUE ("Offset?")) -> ()
                  n96 = Get Date/Time In Seconds() -> (seconds since 1Jan1904=→"Start time":timestamp)
                }
              }
            }
            frame "Process", Default {
              # "Converted to pA"
              # "Magnetic Field"
              # "IV converter"
              # "Elapsed Time"
              n97 = local read "DaQ"() -> (w283:bool)
              n98 = local read "Start time"() -> (w317:timestamp)
              n99 = Unbundle(w319) -> ("seconds since 1Jan1904"=w318:timestamp, "read buffer"=w284:string, "read buffer"=w301:string, "Output"=w281:dbl)
              n100 = local read "B/V (T/V)"() -> (w291:dbl)
              n101 = case shown="False" w283 {
                tunnel: w284 -> [w323 _]
                tunnel: [w322 w324] -> w282
                tunnel: w281 -> [_ w324]
                frame False {
                  n102 = Fract/Exp String To Number(string=w323) -> (number=w322:dbl)  [unwired: 3 in, 1 out]
                }
                frame True {
                }
              }
              n103 = Fract/Exp String To Number(string=w301) -> (number=w311:dbl)  [unwired: 3 in, 1 out]
              n104 = Subtract(x=w318, y=w317) -> (x-y=w296:dbl)
              n105 = Divide(x="Gain (V/A)", y=1000000000000.0) -> (x/y=w294:dbl)
              n106 = Divide(x=w282, y=w294) -> (x/y=w289:dbl)
              n107 = Subtract(x=w296, y=w295) -> (x-y=→"Time Lag":dbl)
              n108 = Build Array (concatenate)(w309, w296) -> (w316:dbl[])
              "Elapsed Time (s)" <- w316
              n109 = local read "Dc offset"() -> (w287:dbl)
              n110 = Subtract(x=w289, y=w287) -> (x-y=w288:dbl)
              "Actual Current (pA)" <- w288
              n111 = Build Array (concatenate)(w314, w288) -> (w315:dbl[])
              "Measured Current (pA)" <- w315
              n112 = local read "B0 (T)"() -> (w290:dbl)
              n113 = xnode "B(U) conversion"("V"=w311, "BpV"=w291, "B0"=w290) -> ("Result"=w310:dbl)  [unwired: 1 in, 1 out]
              "Actual B Field (T)" <- w310
              n114 = Build Array (concatenate)(w312, w310) -> (w313:dbl[])
              "Magnetic Field (T)" <- w313
              n115 = Quotient & Remainder(x=w296, y="Temp Refresh (s)") -> (floor(x/y)=w308:dbl)  [unwired: 1 out]
              n116 = Greater?(x=w308, y=w307) -> (0:w306:bool)
              "Read?" <- w306
              n117 = case shown="True" w306 {
                tunnel: [w328 w353] -> w303
                tunnel: w300 -> [w329 w352]
                tunnel: [w329 w332] -> w299
                tunnel: T6 {"Com Port"=1, "ISOBUS Address"=0, "GPIB Address"=25, "Communication"=enum."GPIB"} ("Address") -> [_ w351]
                tunnel: [w327 w347] -> w285
                frame False {
                  n118 = local read "Setpoint Temperature (K)"() -> (w327:dbl)
                  n119 = local read "Actual Temperature (K)"() -> (w328:dbl)
                }
                frame True {
                  w348 = u32 1000 ("byte count")
                  # "Temperature/Magnet read"
                  n120 = local read "Lock_in_Amplifier"() -> (w336:refnum<visa-resource-name>)
                  n121 = local read "Lake Shore"() -> (w350:refnum<visa-resource-name>)
                  n122 = local read "Magnet"() -> (w339:bool)
                  n123 = case shown="False" w339 {
                    tunnel: w351 -> [_ w357]
                    frame False {
                    }
                    frame True {
                      n124 = call "GPIB - BusCommand.vi"("Command"="R7" ("format string"), "Address"=w357) -> ("Reply"=w358:string)  [unwired: 1 out]
                      n125 = Scan From String(format string="R%f" ("remaining string"), input string=w358) -> (output 1=w356:dbl)  [unwired: 3 in, 3 out]
                      n126 = local write "Actual Field (T)"(w356) -> ()
                    }
                  }
                  n127 = VISA Write(VISA resource name=w350, write buffer="KRDG?a", error in (no error)=w352) -> (VISA resource name out=w346:refnum<visa-resource-name>, error out=w344:errorcluster)  [unwired: 1 out]
                  n128 = VISA Read(VISA resource name=w346, byte count=w348, error in (no error)=w344) -> (VISA resource name out=w345:refnum<visa-resource-name>, read buffer=w354:string, error out=w343:errorcluster)  [unwired: 1 out]
                  n129 = VISA Write(VISA resource name=w345, write buffer="SETP?a", error in (no error)=w343) -> (VISA resource name out=w341:refnum<visa-resource-name>, error out=w342:errorcluster)  [unwired: 1 out]
                  n130 = Fract/Exp String To Number(string=w354) -> (number=w353:dbl)  [unwired: 3 in, 1 out]
                  n131 = VISA Read(VISA resource name=w341, byte count=w348, error in (no error)=w342) -> (read buffer=w340:string, error out=w338:errorcluster)  [unwired: 2 out]
                  n132 = VISA Write(VISA resource name=w336, write buffer="OUTP? 3", error in (no error)=w338) -> (VISA resource name out=w335:refnum<visa-resource-name>, error out=w337:errorcluster)  [unwired: 1 out]
                  n133 = VISA Read(VISA resource name=w335, byte count=u32 1000, error in (no error)=w337) -> (read buffer=w331:string, error out=w332:errorcluster)  [unwired: 2 out]
                  n134 = Fract/Exp String To Number(string=w331) -> (number=→"LockInR":dbl)  [unwired: 3 in, 1 out]
                  n135 = Fract/Exp String To Number(string=w340) -> (number=w347:dbl)  [unwired: 3 in, 1 out]
                }
              }
              "Actual Temperature (K)" <- w303
              "Setpoint Temperature (K)" <- w285
              n136 = Build Array (concatenate)(w305, w303) -> (w304:dbl[])
              "Temperature array" <- w304
              n137 = case shown="True" "Sweep" {
                tunnel: [Mode."Plot" ("Enum") Mode."Sweep" ("Enum")] -> w302
                frame False {
                }
                frame True {
                }
              }
            }
            frame "Sweep" {
              n138 = local read "Temp/Magnetic Field"() -> (w374:bool)
              n139 = case shown="True" w374 {
                tunnel: w384 -> [w393 w450]
                tunnel: [w392 w449] -> w383
                frame False {
                  n140 = local read "Actual Field (T)"() -> (w388:dbl)
                  n141 = local read "Min Field (T)"() -> (w387:dbl)
                  n142 = local read "Max Field (T)"() -> (w394:dbl)
                  n143 = local read "Read?"() -> (w391:bool)
                  n144 = Greater Or Equal?(x=w387, y=w388) -> (x >= y?=w390:bool)
                  n145 = Compound Arithmetic op=AND(w390, w391) -> (w389:bool)
                  n146 = case shown="True" w389 {
                    tunnel: [w397 w433] -> w392
                    tunnel: w394 -> [w395 w432]
                    tunnel: w387 -> [_ w431]
                    tunnel: w388 -> [_ w429]
                    tunnel: w393 -> [w398 w428]
                    frame True {
                      # "Ramp Up"
                      n147 = case shown="True" "First?" {
                        tunnel: [TRUE ("Save") FALSE ("Save")] -> w401
                        tunnel: [w420 w424] -> w400
                        frame False {
                          n148 = local read "Counter"() -> (w423:i8)
                          n149 = local write "Actual Polarization"(0.0 ("Actual Polarization")) -> ()
                          n150 = Increment(x=w423) -> (x+1=w420:i8)
                          n151 = local write "Counter"(w420) -> ()
                        }
                        frame True {
                          n152 = local read "Counter"() -> (w424:i8)
                          n153 = local write "First?"(FALSE ("First?")) -> ()
                        }
                      }
                      "Reset" <- w401
                      n154 = local write "Read?"(FALSE ("Read?")) -> ()
                      n155 = local read "Record ALL"() -> (w396:bool)
                      n156 = case shown="True" w396 {
                        tunnel: w400 -> [_ w408]
                        tunnel: [FALSE w406] -> w399
                        frame False {
                        }
                        frame True {
                          n157 = Greater?(x=w408, y="Max Countl") -> (0:w406:bool)
                        }
                      }
                      n158 = case shown="False" w399 {
                        tunnel: w398 -> [w412 w419]
                        tunnel: [w411 w419] -> w397
                        tunnel: w395 -> [w410 _]
                        frame False {
                          n159 = local read "Magnet"() -> (w409:bool)
                          n160 = case shown="True" w409 {
                            tunnel: w412 -> [w413 w416]
                            tunnel: [w413 w415] -> w411
                            tunnel: w410 -> [_ w414]
                            frame False {
                            }
                            frame True {
                              n161 = call "Set_B.vi"("error in (no error)"=w416, "address string"="25", "Set Field (T)"=w414) -> ("error out"=w415:errorcluster)  [unwired: 8 in]
                            }
                          }
                          "Target Field" <- w410
                        }
                        frame True {
                          "New" <- TRUE
                        }
                      }
                      "Up/Down" <- FALSE ("Up/Down")
                    }
                    frame False {
                      n162 = Less Or Equal?(x=w432, y=w429) -> (x <= y?=w430:bool)
                      n163 = case shown="True" w430 {
                        tunnel: [w434 w438] -> w433
                        tunnel: w431 -> [_ w436]
                        tunnel: w428 -> [w434 w439]
                        frame False {
                        }
                        frame True {
                          # "Resetting at the end of every cycle"
                          # "Ramp Dn"
                          n164 = local write "Up/Down"(TRUE ("Up/Down")) -> ()
                          n165 = local read "Magnet"() -> (w435:bool)
                          n166 = local write "Target Field"(w436) -> ()
                          n167 = local write "Reset"(TRUE ("Reset")) -> ()
                          n168 = case shown="True" w435 {
                            tunnel: w439 -> [w441 w444]
                            tunnel: [w441 w443] -> w438
                            tunnel: w436 -> [_ w442]
                            frame False {
                            }
                            frame True {
                              n169 = call "Set_B.vi"("error in (no error)"=w444, "address string"="25", "Set Field (T)"=w442) -> ("error out"=w443:errorcluster)  [unwired: 8 in]
                            }
                          }
                        }
                      }
                      n170 = local write "Read?"(FALSE ("Read?")) -> ()
                    }
                  }
                }
                frame True {
                  n171 = local read "Setpoint Temperature (K)"() -> (w448:dbl)
                  n172 = local read "Min Temperature (K)"() -> (w447:dbl)
                  n173 = local read "Read?"() -> (w453:bool)
                  n174 = local read "Max temperature (K)"() -> (w446:dbl)
                  n175 = Equal?(x=w448, y=w447) -> (x = y?=w451:bool)
                  n176 = And(x=w451, y=w453) -> (x .and. y?=w452:bool)
                  n177 = case shown="False" w452 {
                    tunnel: [w455 w472] -> w449
                    tunnel: w446 -> [w454 w471]
                    tunnel: w447 -> [_ w470]
                    tunnel: w448 -> [_ w468]
                    tunnel: w450 -> [w456 w467]
                    frame True {
                      # "Ramp Up"
                      n178 = local read "First?"() -> (w462:bool)
                      n179 = case shown="False" w462 {
                        frame False {
                          n180 = local read "Counter"() -> (w465:i8)
                          n181 = Increment(x=w465) -> (x+1=w464:i8)
                          n182 = local write "Counter"(w464) -> ()
                        }
                        frame True {
                        }
                      }
                      n183 = local write "Read?"(FALSE ("Read?")) -> ()
                      n184 = Number To Fractional String(number=w454, precision (6)=i16 3) -> (F-format string=w459:string)  [unwired: 2 in]
                      n185 = local read "Lake Shore"() -> (w457:refnum<visa-resource-name>)
                      n186 = Concatenate Strings("SETP 1," ("write buffer"), w459) -> (w461:string)
                      n187 = VISA Write(VISA resource name=w457, write buffer=w461, error in (no error)=w456) -> (error out=w455:errorcluster)  [unwired: 2 out]
                    }
                    frame False {
                      n188 = Equal?(x=w471, y=w468) -> (x = y?=w469:bool)
                      n189 = case shown="True" w469 {
                        tunnel: [w473 w476] -> w472
                        tunnel: w470 -> [_ w475]
                        tunnel: w467 -> [w473 w477]
                        frame False {
                        }
                        frame True {
                          # "Ramp Dn"
                          n190 = local write "Up/Down"(TRUE ("Up/Down")) -> ()
                          n191 = Number To Fractional String(number=w475, precision (6)=i16 3) -> (F-format string=w479:string)  [unwired: 2 in]
                          n192 = local read "Lake Shore"() -> (w474:refnum<visa-resource-name>)
                          n193 = Concatenate Strings("SETP 1," ("write buffer"), w479) -> (w481:string)
                          n194 = VISA Write(VISA resource name=w474, write buffer=w481, error in (no error)=w477) -> (error out=w476:errorcluster)  [unwired: 2 out]
                        }
                      }
                      n195 = local write "Read?"(FALSE ("Read?")) -> ()
                    }
                  }
                }
              }
              n196 = local read "Magnet"() -> (w373:bool)
              n197 = case shown="False" w373 {
                tunnel: [Mode."StepDelta" ("Enum") Mode."Plot" ("Enum")] -> w375
                frame False {
                }
                frame True {
                }
              }
            }
            frame "StepDelta" {
              n198 = flat-sequence {
                tunnel: w484 -> [w500]
                tunnel: [w499] -> w483
                frame #0 {
                  # "Check if it is time to step Field"
                  n199 = local read "Sweep Rate (T/min)"() -> (w501:dbl)
                  n200 = local read "B/V (T/V)"() -> (w493:dbl)
                  n201 = local read "Time Lag"() -> (w497:dbl)
                  n202 = xnode "Sweep Delay"("SweepRate"=w501, "Resolution"=0.001 ("Voltage Step (V)"), "BpV"=w493) -> ("Result"=w498:dbl)  [unwired: 1 in, 1 out]
                  n203 = Divide(x=w497, y=w498) -> (x/y=w495:dbl)
                  n204 = Multiply(x=0.001 ("y"), y=w495) -> (x*y=w494:dbl)
                  "deltaUaux" <- w494
                  n205 = stacked-sequence {
                    tunnel: w500 -> [_ w525]
                    tunnel: [_ w524] -> w499
                    tunnel: w494 -> [w503 _]
                    frame #0 {
                      n206 = local read "Actual Voltage (V)"() -> (w508:dbl)
                      n207 = local read "Up/Down"() -> (w509:bool)
                      n208 = Add(x=w508, y=w503) -> (x+y=w505:dbl)
                      n209 = Subtract(x=w508, y=w503) -> (x-y=w504:dbl)
                      n210 = Select(t=w504, s=w509, f=w505) -> (s? t:f=w507:dbl)
                      "Actual Voltage (V)" <- w507
                      n211 = local read "V/I (Ohm)"() -> (w510:dbl)
                      n212 = local read "B/V (T/V)"() -> (w511:dbl)
                      n213 = xnode "AUXtoB"("BpV"=w511, "Rm"=w510, "Aux"=w507) -> ("Result"=w506:dbl)  [unwired: 1 in, 1 out]
                      n214 = local write "Actual Field (T)"(w506) -> ()
                    }
                    frame #1 {
                      n215 = local read "Actual Voltage (V)"() -> (w530:dbl)
                      n216 = local read "Lock_in_Amplifier"() -> (w526:refnum<visa-resource-name>)
                      n217 = Format Into String(w530) -> (resulting string=w529:string)  [unwired: 3 in, 1 out]
                      n218 = Concatenate Strings("AUXV 1,", w529) -> (w527:string)
                      n219 = VISA Write(VISA resource name=w526, write buffer=w527, error in (no error)=w525) -> (error out=w524:errorcluster)  [unwired: 2 out]
                    }
                  }
                }
              }
            }
            frame "Plot" {
              # "dI"
              n220 = local read "P(uC/mm^2)"() -> (w544:dbl[])
              n221 = local read "Actual Polarization"() -> (w543:dbl)
              n222 = local read "Actual Current (pA)"() -> (w545:dbl)
              n223 = local read "Time Lag"() -> (w557:dbl)
              n224 = Multiply(x=w545, y=w557) -> (x*y=w549:dbl)
              n225 = Divide(x=w549, y="Sample area (mm^2)") -> (x/y=w548:dbl)
              n226 = Add(x=w548, y=w543) -> (x+y=w547:dbl)
              "Actual Polarization" <- w547
              n227 = local read "Temp/Magnetic Field"() -> (w558:bool)
              n228 = Build Array (concatenate)(w544, w547) -> (→"P(uC/mm^2)":dbl[])
              n229 = case shown="False" w558 {
                tunnel: w555 -> [_ w618]
                tunnel: w552 -> [_ w600]
                tunnel: w547 -> [w565 w601]
                frame False {
                  # "Magnetic Field plotting"
                  n230 = local read "Up/Down"() -> (w570:bool)
                  n231 = case shown="True" w570 {
                    frame True {
                      # "Down"
                      n232 = local read "I(B) 3"() -> (w580:cluster{dbl[], dbl[]}[])
                      n233 = local read "I(B) 3"() -> (w584:cluster{dbl[], dbl[]}[])
                      n234 = Index Array(array=w580, index=1) -> (element=w578:cluster{dbl[], dbl[]})
                      n235 = Unbundle(w578) -> (w577:dbl[], w576:dbl[])
                      n236 = Index Array(array=w584, index=i8 0 ("t")) -> (element=w581:cluster{dbl[], dbl[]})
                      n237 = local read "Actual Current (pA)"() -> (w571:dbl)
                      n238 = local read "Actual B Field (T)"() -> (w573:dbl)
                      n239 = Build Array (concatenate)(w577, w573) -> (w575:dbl[])
                      n240 = Build Array (concatenate)(w576, w571) -> (w574:dbl[])
                      n241 = Bundle(w575, w574) -> (w572:cluster{dbl[], dbl[]})  [unwired: 1 in]
                      n242 = Build Array(w581, w572) -> (w582:cluster{dbl[], dbl[]}[])
                      n243 = local write "I(B) 3"(w582) -> ()
                    }
                    frame False {
                      # "Up"
                      n244 = local read "I(B) 3"() -> (w596:cluster{dbl[], dbl[]}[])
                      n245 = local read "I(B) 3"() -> (w598:cluster{dbl[], dbl[]}[])
                      n246 = Index Array(array=w596, index=0) -> (element=w594:cluster{dbl[], dbl[]})
                      n247 = Unbundle(w594) -> (w593:dbl[], w592:dbl[])
                      n248 = Index Array(array=w598, index=i8 1 ("t")) -> (element=w587:cluster{dbl[], dbl[]})
                      n249 = local read "Actual B Field (T)"() -> (w588:dbl)
                      n250 = Build Array (concatenate)(w593, w588) -> (w591:dbl[])
                      n251 = local read "Actual Current (pA)"() -> (w585:dbl)
                      n252 = Build Array (concatenate)(w592, w585) -> (w590:dbl[])
                      n253 = Bundle(w591, w590) -> (w589:cluster{dbl[], dbl[]})  [unwired: 1 in]
                      n254 = Build Array(w589, w587) -> (w586:cluster{dbl[], dbl[]}[])
                      n255 = local write "I(B) 3"(w586) -> ()
                    }
                  }
                  n256 = local read "Actual B Field (T)"() -> (w567:dbl)
                  n257 = local read "P(B)"() -> (w569:cluster{"yi":dbl[], dbl[]})
                  n258 = Unbundle(w569) -> ("yi"=w568:dbl[], w566:dbl[])
                  n259 = Build Array (concatenate)(w568, w567) -> (w564:dbl[])
                  n260 = Build Array (concatenate)(w566, w565) -> (w563:dbl[])
                  n261 = Bundle(w564, w563) -> (→"P(B)":cluster{dbl[], dbl[]})  [unwired: 1 in]
                }
                frame True {
                  # "Temperature plotting"
                  n262 = Quotient & Remainder(x=w618, y="Save Period") -> (x-y*floor(x/y)=w599:dbl)  [unwired: 1 out]
                  n263 = Greater?(x=w600, y=w599) -> (0:w616:bool)
                  n264 = local read "Actual Temperature (K)"() -> (w603:dbl)
                  n265 = local read "Actual Current (pA)"() -> (w609:dbl)
                  n266 = local read "P(T)"() -> (w605:cluster{"yi":dbl[], dbl[]})
                  n267 = local read "I(T)"() -> (w615:cluster{dbl[], dbl[]})
                  n268 = case shown="True" w616 {
                    frame False {
                    }
                    frame True {
                      n269 = local write "Reset"(TRUE) -> ()
                    }
                  }
                  n270 = Unbundle(w605) -> ("yi"=w606:dbl[], w602:dbl[])
                  n271 = Unbundle(w615) -> (w613:dbl[], w612:dbl[])
                  n272 = Build Array (concatenate)(w606, w603) -> (w607:dbl[])
                  n273 = Build Array (concatenate)(w602, w601) -> (w608:dbl[])
                  n274 = Build Array (concatenate)(w613, w603) -> (w611:dbl[])
                  n275 = Build Array (concatenate)(w612, w609) -> (w610:dbl[])
                  n276 = Bundle(w611, w610) -> (→"I(T)":cluster{dbl[], dbl[]})  [unwired: 1 in]
                  n277 = Bundle(w607, w608) -> (→"P(T)":cluster{dbl[], dbl[]})  [unwired: 1 in]
                }
              }
            }
            frame "Save" {
              n278 = local read "Reset"() -> (w620:bool)
              n279 = case shown="True" w620 {
                tunnel: w625 -> [w642 w644]
                tunnel: [w642 w647] -> w630
                tunnel: w624 -> [w641 w645]
                tunnel: [w641 w647] -> w629
                tunnel: w626 -> [w640 w646]
                tunnel: [w640 w647] -> w628
                tunnel: [w639 w647] -> w627
                tunnel: w623 -> [w639 w643]
                frame False {
                }
                frame True {
                  n280 = stacked-sequence {
                    tunnel: [_ _ w698] -> w647
                    tunnel: w646 -> [_ w687 _]
                    tunnel: w645 -> [w673 w685 _]
                    tunnel: w644 -> [w674 w686 _]
                    tunnel: w643 -> [w664 w683 _]
                    frame #0 {
                      n281 = local read "B array"() -> (w658:dbl[])
                      n282 = local read "Counter"() -> (w672:i8)
                      n283 = local read "Averaged I(B)"() -> (w649:dbl[][])
                      n284 = local read "Up/Down"() -> (w675:bool)
                      n285 = local read "Sample area (mm^2)"() -> (w654:dbl)
                      n286 = call "Average_IBP_curves_baseline.vi"("I in"=w673, "Averaged P(B) In"="Averaged P(B)", "Counter"=w672, "B0"="Threshold B (T)", "Averaged I(B) In"=w649, "t in"=w664, "B in"=w674, "Averaged dt in"="Averaged dt", "Up/Down"=w675, "Sample area(mm^2)"=w654, "B array"=w658) -> ("Averaged dt Out"=w661:dbl[][], "Averaged P(B) Out"=w650:dbl[][], "BaselineSubtracted I(B)"=w648:dbl[][])  [unwired: 1 in, 1 out]
                      "Averaged I(B)" <- w648
                      n287 = Index Array(array=w650, index (row)=0 ("disabled index (col)")) -> (element=w659:dbl[])  [unwired: 1 in]
                      n288 = Index Array(array=w650, index (row)=1 ("disabled index (col)")) -> (element=w660:dbl[])  [unwired: 1 in]
                      n289 = Index Array(array=w648, index (row)=0 ("disabled index (col)")) -> (element=w666:dbl[])  [unwired: 1 in]
                      n290 = Index Array(array=w648, index (row)=1 ("disabled index (col)")) -> (element=w665:dbl[])  [unwired: 1 in]
                      n291 = local write "Averaged dt"(w661) -> ()
                      n292 = Bundle("B array"=w658, "Averaged P(B) Out"=w659) -> (w657:T7)  [unwired: 1 in]
                      n293 = Bundle("B array"=w658, "Averaged P(B) Out"=w660) -> (w656:T7)  [unwired: 1 in]
                      n294 = local write "Averaged P(B)"(w650) -> ()
                      n295 = Bundle("B array"=w658, "BaselineSubtracted I(B)"=w666) -> (w671:T8)  [unwired: 1 in]
                      n296 = Bundle("B array"=w658, "BaselineSubtracted I(B)"=w665) -> (w670:T8)  [unwired: 1 in]
                      n297 = Build Array(w657, w656) -> (→"P(B) /Averaged/":T9)
                      n298 = Build Array(w671, w670) -> (→"I(B) /Averaged/":T10)
                    }
                    frame #1 {
                      # "Save and Reset"
                      n299 = local read "Temp/Magnetic Field"() -> (w676:bool)
                      n300 = local read "Measurement File"() -> (w678:path)
                      n301 = local read "P(uC/mm^2)"() -> (w684:dbl[])
                      n302 = Build Array(w687, w686, w685, w683, w684) -> (w677:dbl[][])
                      n303 = case shown="False" w676 {
                        tunnel: w678 -> [_ _]
                        tunnel: w677 -> [w692 _]
                        frame False {
                          n304 = local read "Up/Down"() -> (w690:bool)
                          n305 = case shown="False" w690 {
                            tunnel: [w695 w696] -> w689
                            frame False {
                              n306 = local read "Measurement File_dn"() -> (w695:path)
                            }
                            frame True {
                              n307 = local read "Measurement File_up"() -> (w696:path)
                            }
                          }
                          n308 = call-poly <vilib>:"Write Delimited Spreadsheet.vi"("file path (dialog if empty)"=w689, "format (%.3f)"="%.5g", "2D data"=w692, "append to file? (F)"=TRUE ("transpose? (F)"), "transpose? (F)"=FALSE ("append to file? (F)")) -> ()  [unwired: 9 in, 2 out]
                        }
                        frame True {
                        }
                      }
                      n309 = case shown="False" "Reset IB?" {
                        frame False {
                        }
                        frame True {
                          n310 = local read "Up/Down"() -> (w697:bool)
                          n311 = case shown="False" w697 {
                            frame False {
                              n312 = invoke on="I(B) 3" class="XYGraph (strict)" method="Reinit To Default"() -> ()  [unwired: 3 in, 3 out]
                            }
                            frame True {
                            }
                          }
                        }
                      }
                      n313 = call-poly <vilib>:"Write Delimited Spreadsheet.vi"("file path (dialog if empty)"=w678, "format (%.3f)"="%.5g", "2D data"=w677, "append to file? (F)"=TRUE, "transpose? (F)"=TRUE) -> ()  [unwired: 9 in, 2 out]
                      n314 = local write "Reset"(FALSE ("Save")) -> ()
                    }
                    frame #2 {
                      w698 = dbl[] []
                      n315 = local write "P(uC/mm^2)"(w698) -> ()
                    }
                  }
                }
              }
              n316 = local read "New"() -> (w622:bool)
              n317 = case shown="True" w622 {
                tunnel: [Mode."Return" ("Enum") Mode."New" ("Enum")] -> w634
                tunnel: [TRUE FALSE] -> w621
                frame False {
                }
                frame True {
                }
              }
            }
            frame "New" {
              n318 = stacked-sequence {
                seq-local: [_ _ _ _ w800 _ _] -> [_ _ _ _ _ w809 _]
                seq-local: [_ _ w754 _ _ _ _] -> [_ _ _ _ w799 _ _]
                tunnel: T6 {"Com Port"=1, "ISOBUS Address"=0, "GPIB Address"=25, "Communication"=enum."GPIB"} ("Address") -> [_ _ w753 w794 _ _ _]
                tunnel: w701 -> [_ _ w755 _ _ w810 _]
                tunnel: [_ _ _ _ _ w812 _] -> w700
                tunnel: w699 -> [_ w734 _ _ _ _ _]
                frame #0 {
                  w727 = 1 ("index (row)")
                  w726 = 0 ("index (row)")
                  # "Save averages"
                  n319 = local read "Measurement File_average"() -> (w714:path)
                  n320 = local read "Averaged P(B)"() -> (w725:dbl[][])
                  n321 = local read "Averaged dt"() -> (w723:dbl[][])
                  n322 = local read "I(B) /Averaged/"() -> (w715:cluster{"B array":dbl[], dbl[]}[])
                  n323 = Index Array(array=w723, index (row)=w726) -> (element=w724:dbl[])  [unwired: 1 in]
                  n324 = Index Array(array=w723, index (row)=w727) -> (element=w731:dbl[])  [unwired: 1 in]
                  n325 = Index Array(array=w715, index=1) -> (element=w719:cluster{"B array":dbl[], dbl[]})
                  n326 = Index Array(array=w715, index=0) -> (element=w718:cluster{"B array":dbl[], dbl[]})
                  n327 = Unbundle(w719) -> ("B array"=w729:dbl[], w730:dbl[])
                  n328 = Unbundle(w718) -> ("B array"=w720:dbl[], w721:dbl[])
                  n329 = Index Array(array=w725, index (row)=w726) -> (element=w728:dbl[])  [unwired: 1 in]
                  n330 = Index Array(array=w725, index (row)=w727) -> (element=w732:dbl[])  [unwired: 1 in]
                  n331 = Build Array(w720, w721, w724, w728, w729, w730, w731, w732) -> (w722:dbl[][])
                  n332 = call-poly <vilib>:"Write Delimited Spreadsheet.vi"("file path (dialog if empty)"=w714, "format (%.3f)"="%.5g", "2D data"=w722, "append to file? (F)"=TRUE ("transpose? (F)"), "transpose? (F)"=TRUE ("append to file? (F)")) -> ()  [unwired: 9 in, 2 out]
                }
                frame #1 {
                  w740 = dbl[] []
                  w749 = dbl[] []
                  # "Reset Flags"
                  n333 = Get Date/Time In Seconds() -> (seconds since 1Jan1904=w750:timestamp)
                  n334 = local write "Up/Down"(TRUE ("Up/Down")) -> ()
                  n335 = local write "First?"(TRUE ("First?")) -> ()
                  n336 = local write "Offset?"(FALSE ("Offset?")) -> ()
                  n337 = local write "New"(FALSE ("New")) -> ()
                  n338 = local write "P(uC/mm^2)"(w749) -> ()
                  n339 = local write "Start time"(w750) -> ()
                  n340 = local write "Offset array"(w749) -> ()
                  n341 = local write "Actual Polarization"(0.0 ("Actual Polarization")) -> ()
                  n342 = local write "Up/Down"(TRUE ("Up/Down")) -> ()
                  n343 = local write "Reset"(FALSE ("Reset")) -> ()
                  n344 = local read "B array"() -> (w743:dbl[])
                  n345 = local write "Counter"(i8 0 ("Counter")) -> ()
                  n346 = invoke on="P(B)" class="XYGraph (strict)" method="Reinit To Default"() -> ()  [unwired: 3 in, 3 out]
                  n347 = invoke on="I(B) 3" class="XYGraph (strict)" method="Reinit To Default"() -> ()  [unwired: 3 in, 3 out]
                  n348 = Multiply(x=w743, y=0.0) -> (x*y=w744:dbl[])
                  n349 = Build Array(w740, w740) -> (w748:dbl[][])
                  n350 = Bundle("B array"=w743, w744) -> (w745:cluster{"B array":dbl[], dbl[]})  [unwired: 1 in]
                  n351 = local write "Averaged I(B)"(w748) -> ()
                  n352 = Build Array(w745, w745) -> (w746:cluster{"B array":dbl[], dbl[]}[])
                  n353 = local write "I(B) /Averaged/"(w746) -> ()
                  n354 = local write "Measuring"(FALSE ("Measuring")) -> ()
                  n355 = Flush Queue(queue=w734) -> (remaining elements=→"remaining elements 2":T1)  [unwired: 1 in, 2 out]
                }
                frame #2 {
                  # "Step"
                  n356 = local read "Sweep Rate Array"() -> (w759:dbl[])
                  n357 = local read "j"() -> (w760:i32)
                  n358 = Increment(x=w760) -> (x+1=w756:i32)
                  n359 = Array Size(array=w759) -> (size(s)=w758:i32)
                  n360 = Less?(x=w756, y=w758) -> (x < y?=w757:bool)
                  "Step Rate" <- w757
                  n361 = case shown="True" w757 {
                    tunnel: w756 -> [_ w787]
                    tunnel: w755 -> [w763 w786]
                    tunnel: [w762 w786] -> w754
                    tunnel: w753 -> [w761 _]
                    frame False {
                      # "Step Temp?"
                      n362 = local read "Temperature Array"() -> (w767:dbl[])
                      n363 = local read "i"() -> (w768:i32)
                      n364 = Increment(x=w768) -> (x+1=w765:i32)
                      n365 = local write "j"(0 ("f")) -> ()
                      n366 = Array Size(array=w767) -> (size(s)=w766:i32)
                      n367 = Less?(x=w765, y=w766) -> (x < y?=w764:bool)
                      "Step Temp" <- w764
                      n368 = case shown="False" w764 {
                        tunnel: w765 -> [_ w785]
                        tunnel: w763 -> [w773 w784]
                        tunnel: [w772 w784] -> w762
                        tunnel: w761 -> [w771 _]
                        frame False {
                          # "Heater OFF"
                          # "Finished"
                          n369 = local write "i"(0 ("i")) -> ()
                          n370 = stacked-sequence {
                            tunnel: w773 -> [w777 _ _]
                            tunnel: [w776 _ _] -> w772
                            tunnel: w771 -> [_ w781 w782]
                            frame #0 {
                              n371 = local read "Lake Shore"() -> (w778:refnum<visa-resource-name>)
                              n372 = VISA Write(VISA resource name=w778, write buffer="RANGE,1,0", error in (no error)=w777) -> (error out=w776:errorcluster)  [unwired: 2 out]
                            }
                            frame #1 {
                              n373 = call "ips_switchHeaterOff.vi"("Instrument address"=w781, "Rate"=2.0) -> ()  [unwired: 1 out]
                            }
                            frame #2 {
                              n374 = call "GPIB - BusCommand.vi"("Command"="H0", "Address"=w782) -> ()  [unwired: 2 out]
                            }
                          }
                          n375 = local write "Record ALL"(FALSE ("Record ALL")) -> ()
                          "Finished" <- TRUE
                        }
                        frame True {
                          n376 = local write "i"(w785) -> ()
                        }
                      }
                    }
                    frame True {
                      n377 = local write "j"(w787) -> ()
                    }
                  }
                }
                frame #3 {
                  # "Set rates"
                  n378 = local read "Sweep Rate Array"() -> (w793:dbl[])
                  n379 = local read "j"() -> (w792:i32)
                  n380 = local read "j"() -> (w790:i32)
                  n381 = Index Array(array=w793, index=w792) -> (element=w791:dbl)
                  n382 = Number To Fractional String(number=w791, precision (6)=i16 3) -> (F-format string=w797:string)  [unwired: 2 in]
                  n383 = Index Array(array="Max count array", index=w790) -> (element=w788:i32)
                  n384 = local write "Max Countl"(w788) -> ()
                  n385 = Concatenate Strings("T" ("format string"), w797) -> (w798:string)
                  n386 = call "GPIB - BusCommand.vi"("Command"=w798, "Address"=w794) -> ()  [unwired: 2 out]
                  n387 = local write "Sweep Rate (T/min)"(w791) -> ()
                }
                frame #4 {
                  # "Set temperature"
                  n388 = local read "Temperature Array"() -> (w803:dbl[])
                  n389 = local read "i"() -> (w802:i32)
                  n390 = Index Array(array=w803, index=w802) -> (element=w801:dbl)
                  n391 = local read "Lake Shore"() -> (w805:refnum<visa-resource-name>)
                  n392 = Number To Fractional String(number=w801, precision (6)=i16 3) -> (F-format string=w806:string)  [unwired: 2 in]
                  n393 = Concatenate Strings("SETP 1," ("write buffer"), w806) -> (w808:string)
                  n394 = VISA Write(VISA resource name=w805, write buffer=w808, error in (no error)=w799) -> (error out=w800:errorcluster)  [unwired: 2 out]
                }
                frame #5 {
                  n395 = local read "Finished"() -> (w811:bool)
                  n396 = case shown="False" w811 {
                    tunnel: [w825 w862] -> w812
                    tunnel: w810 -> [_ _]
                    tunnel: w809 -> [w822 w862]
                    frame False {
                      w820 = "_" ("string")
                      # "Wait, create Files"
                      n397 = local read "Temperature Array"() -> (w852:dbl[])
                      n398 = local read "Sweep Rate Array"() -> (w848:dbl[])
                      n399 = local read "i"() -> (w851:i32)
                      n400 = local read "j"() -> (w849:i32)
                      n401 = Index Array(array=w852, index=w851) -> (element=w850:dbl)
                      n402 = Index Array(array=w848, index=w849) -> (element=w817:dbl)
                      n403 = Round Toward -Infinity(1:w817) -> (0:w818:dbl)
                      n404 = Number To Fractional String(use system decimal point (T)=TRUE, number=w850, precision (6)=i16 1) -> (F-format string=w853:string)  [unwired: 1 in]
                      n405 = Subtract(x=w817, y=w818) -> (x-y=w819:dbl)
                      n406 = Equal To 0?(x=w819) -> (x = 0?=w816:bool)
                      n407 = Select(t=i16 0 ("precision (6)"), s=w816, f=i16 2 ("precision (6)")) -> (s? t:f=w813:i16)
                      n408 = Number To Fractional String(use system decimal point (T)=TRUE, number=w817, precision (6)=w813) -> (F-format string=w821:string)  [unwired: 1 in]
                      n409 = Concatenate Strings("Directory", "\\" ("string"), "FileName", w820, w853, "K" ("string"), w820, w821, "Tpm" ("string")) -> (w842:string)
                      n410 = Search and Replace String(replace all?=TRUE ("replace all? (F)"), input string=w842, search string=".", replace string="p" ("substring (\"\")"), error in=w822) -> (result string=w837:string, error out=w832:errorcluster)  [unwired: 3 in, 2 out]
                      n411 = local write "Step Rate"(FALSE ("Step Rate")) -> ()
                      n412 = Concatenate Strings(w837, ".txt" ("string")) -> (w836:string)
                      n413 = local read "Step Temp"() -> (w826:bool)
                      n414 = String To Path(string=w836) -> (path=w835:path)
                      n415 = Open/Create/Replace File(file path (use dialog)=w835, error in=w832, operation (0:open)=T5."open or create") -> (refnum out=w824:refnum<file>, error out=w825:errorcluster)  [unwired: 3 in, 1 out]
                      n416 = local write "refnum out"(w824) -> ()
                      n417 = Refnum to Path(1:w824) -> (0:w827:path)
                      n418 = call "Create_sweep_files.vi"("Measurement File"=w827) -> ("Path 3"=w830:path, "Path 2"=w829:path, "Path"=w828:path)  [unwired: 8 in]
                      n419 = local write "Measurement File"(w827) -> ()
                      n420 = case shown="True" w826 {
                        frame False {
                        }
                        frame True {
                          n421 = Get Date/Time In Seconds() -> (seconds since 1Jan1904=w855:timestamp)
                          n422 = local write "Step Temp"(FALSE ("Step Temp")) -> ()
                          n423 = while {
                            tunnel: w855 -> [w860]
                            stop <- w857 stop-if-true
                            n424 = Get Date/Time In Seconds() -> (seconds since 1Jan1904=w861:timestamp)
                            n425 = Subtract(x=w861, y=w860) -> (x-y=w859:dbl)
                            "Wait (s)" <- w859
                            n426 = Greater Or Equal?(x=w859, y="secs to wait") -> (x >= y?=w857:bool)
                          }
                        }
                      }
                      n427 = local write "Measurement File_dn"(w830) -> ()
                      n428 = local write "Measurement File_average"(w828) -> ()
                      n429 = local write "Measurement File_up"(w829) -> ()
                    }
                    frame True {
                    }
                  }
                }
                frame #6 {
                  n430 = local read "Finished"() -> (w863:bool)
                  n431 = case shown="True" w863 {
                    frame False {
                      n432 = local write "Measuring"(TRUE ("Measuring")) -> ()
                    }
                    frame True {
                      n433 = local write "Measure /Pause"(FALSE ("Measure /Pause")) -> ()
                    }
                  }
                }
              }
            }
            frame "Return" {
            }
          }
        }
      }
      frame Error {
        # "Return true for any case which should stop the loop."
      }
    }
  }
  n434 = VISA Read(VISA resource name=w5, byte count=u32 100, error in (no error)=w7) -> (VISA resource name out=w4:refnum<visa-resource-name>, read buffer=w3:string, error out=w6:errorcluster)  [unwired: 1 out]
  n435 = VISA Open(error in (no error)=w6, VISA resource name="Magnetic Field") -> (VISA resource name=w100:refnum<visa-resource-name>, error out=w82:errorcluster)  [unwired: 3 in]
  n436 = VISA Open(error in (no error)=w82, VISA resource name="Lake Shore") -> (VISA resource name=w77:refnum<visa-resource-name>, error out=w46:errorcluster)  [unwired: 3 in]
  n437 = VISA Write(VISA resource name="Lake Shore", write buffer="KRDG?a", error in (no error)=w46) -> (VISA resource name out=w43:refnum<visa-resource-name>, error out=w42:errorcluster)  [unwired: 1 out]
  n438 = VISA Read(VISA resource name=w43, byte count=w49, error in (no error)=w42) -> (VISA resource name out=w40:refnum<visa-resource-name>, read buffer=w54:string, error out=w41:errorcluster)  [unwired: 1 out]
  n439 = VISA Write(VISA resource name=w40, write buffer="SETP?a", error in (no error)=w41) -> (VISA resource name out=w39:refnum<visa-resource-name>, error out=w38:errorcluster)  [unwired: 1 out]
  n440 = VISA Read(VISA resource name=w39, byte count=w49, error in (no error)=w38) -> (VISA resource name out=w36:refnum<visa-resource-name>, read buffer=w53:string, error out=w37:errorcluster)  [unwired: 1 out]
  n441 = VISA Write(VISA resource name=w36, write buffer="RANGE?a", error in (no error)=w37) -> (VISA resource name out=w34:refnum<visa-resource-name>, error out=w35:errorcluster)  [unwired: 1 out]
  n442 = Fract/Exp String To Number(string=w54) -> (number=w52:dbl)  [unwired: 3 in, 1 out]
  n443 = VISA Read(VISA resource name=w34, byte count=w49, error in (no error)=w35) -> (read buffer=w48:string, error out=w45:errorcluster)  [unwired: 2 out]
  n444 = Fract/Exp String To Number(string=w53) -> (number=w51:dbl)  [unwired: 3 in, 1 out]
  n445 = Fract/Exp String To Number(string=w48) -> (number=w44:dbl)  [unwired: 3 in, 1 out]
  n446 = local write "Actual Temperature (K)"(w52) -> ()
  n447 = local write "Setpoint Temperature (K)"(w51) -> ()
  n448 = local write "Heater Range"(w44) -> ()
  n449 = case shown="True" w59 {
    frame False {
    }
    frame True {
      n450 = invoke on="P(T)" class="XYGraph (strict)" method="Reinit To Default"() -> ()  [unwired: 3 in, 3 out]
      n451 = invoke on="I(T)" class="XYGraph (strict)" method="Reinit To Default"() -> ()  [unwired: 3 in, 3 out]
    }
  }
  n452 = Decimal String To Number(string=w3) -> (number=w2:i32)  [unwired: 2 in, 1 out]
  n453 = local write "Keithley (IV conv) averaging"(w2) -> ()
  n454 = while {
    shift-right: [w894] -> w98
    shift-left: w79 -> [w895]
    shift-right: [w896] -> w103
    shift-left: w104 -> [w897]
    tunnel: w4 -> [w893]
    tunnel: w100 -> [w892]
    tunnel: w45 -> [_]
    tunnel: [w886] -> _
    tunnel: w87 -> [w885]
    tunnel: w77 -> [w884]
    tunnel: w12 -> [w883]
    stop <- "stop" stop-if-true
    n455 = event shown="[10] \"Calibrate\": Value Change" {
      selector: _ -> [_ _ _ _ _ _ _ _ _ _ _ _ _ _ _ _]
      dyn-events: _ -> [_ _ _ _ _ _ _ _ _ _ _ _ _ _ _ _]
      timeout: 10 -> [_ _ _ _ _ _ _ _ _ _ _ _ _ _ _ _]
      tunnel: w897 -> [w907 w953 w971 w981 w995 w1066 w1070 w1074 w1114 w1130 w1147 w1190 w1207 w1223 w1233 w1244]
      tunnel: [w906 w953 w971 w981 w995 w1066 w1070 w1074 w1114 w1130 w1147 w1190 w1207 w1223 w1233 w1244] -> w896
      tunnel: w895 -> [w905 w962 w970 w980 w993 w1065 w1072 w1076 w1115 w1129 w1146 w1191 w1209 w1227 w1237 w1246]
      tunnel: [w904 w954 w970 w980 w992 w1067 w1072 w1075 _ w1129 w1146 w1191 w1208 w1226 w1236 w1245] -> w894
      tunnel: w893 -> [w903 w963 _ _ _ _ _ _ _ _ _ _ _ _ _ _]
      tunnel: w892 -> [w902 _ _ _ _ _ _ _ _ _ _ _ _ _ _ _]
      tunnel: [w900 w952 w969 w979 w994 w1068 w1071 w1073 w1113 w1128 w1145 w1189 w1206 w1224 w1234 _] -> w886
      tunnel: w885 -> [w900 w952 w969 w982 w994 w1068 w1071 w1073 w1113 w1128 w1145 w1189 w1206 w1224 w1234 _]
      tunnel: w884 -> [_ _ _ _ _ _ _ _ _ _ _ _ w1210 w1225 w1238 w1243]
      tunnel: [_ _ _ _ _ _ _ _ w1115 _ _ _ _ _ _ _] -> _
      tunnel: w883 -> [w899 _ _ _ _ _ _ _ _ _ _ _ _ _ _ _]
      event Timeout {
        n456 = event-data() -> ()  [unwired: 1 in, 3 out]
        n457 = case shown="True" "Measuring" {
          tunnel: w907 -> [w909 w932]
          tunnel: [w909 w931] -> w906
          tunnel: w905 -> [w908 w910]
          tunnel: [w908 w930] -> w904
          tunnel: w903 -> [_ w923]
          tunnel: w902 -> [_ w922]
          tunnel: w899 -> [_ w913]
          frame False {
          }
          frame True {
            w921 = ":FETCh? " ("data")
            w924 = u32 1000 ("byte count")
            # "Generate the data here."
            n458 = case shown="No Error" w910 {
              selector: w910 -> [w944 w945]
              tunnel: [w944 w945] -> w918
              tunnel: [w943 _] -> w917
              frame No Error {
                n459 = Get Date/Time In Seconds() -> (seconds since 1Jan1904=w943:timestamp)
              }
              frame Error {
              }
            }
            n460 = VISA Write(VISA resource name=w923, write buffer=w921, error in (no error)=w918) -> (VISA resource name out=w929:refnum<visa-resource-name>, error out=w927:errorcluster)  [unwired: 1 out]
            n461 = VISA Write(VISA resource name=w922, write buffer=w921, error in (no error)=w927) -> (VISA resource name out=w928:refnum<visa-resource-name>, error out=w926:errorcluster)  [unwired: 1 out]
            n462 = VISA Read(VISA resource name=w929, byte count=w924, error in (no error)=w926) -> (read buffer=w919:string, error out=w925:errorcluster)  [unwired: 2 out]
            n463 = VISA Read(VISA resource name=w928, byte count=w924, error in (no error)=w925) -> (read buffer=w920:string, error out=w915:errorcluster)  [unwired: 2 out]
            n464 = case shown="True" "DaQ" {
              tunnel: w915 -> [w934 w940]
              tunnel: [w934 w939] -> w914
              tunnel: w913 -> [_ w938]
              tunnel: [0.0 ("Output") w936] -> w911
              frame False {
              }
              frame True {
                n465 = local read "Number of Samples"() -> (w942:i32)
                n466 = call-poly <vilib>:"DAQmx Read.vi"("task/channels in"=w938, "number of samples per channel"=w942, "error in"=w940) -> ("data"=w941:dbl[], "error out"=w939:errorcluster)  [unwired: 10 in, 1 out]
                n467 = call-poly <vilib>:"Mean.vi"("X"=w941) -> ("mean"=w937:dbl)  [unwired: 1 out]
                "Actual mean" <- w937
                n468 = call "N Point Running Average.vi"("n"="Moving average", "Input"=w937) -> ("Output"=w936:dbl)
              }
            }
            n469 = Bundle("seconds since 1Jan1904"=w917, "read buffer"=w919, "read buffer"=w920, "Output"=w911) -> (w916:T4)  [unwired: 1 in]
            n470 = Enqueue Element(queue=w932, element=w916, error in (no error)=w914) -> (queue out=w931:refnum<queue>, error out=w930:errorcluster)  [unwired: 1 in, 1 out]
          }
        }
      }
      event "Keithley (IV conv) averaging": Value Change {
        n471 = event-data() -> ()  [unwired: 1 in, 6 out]
        n472 = Number To Decimal String(number="Keithley (IV conv) averaging") -> (decimal integer string=w960:string)  [unwired: 1 in]
        n473 = Concatenate Strings("VOLTage:DC:AVERage:COUNt " ("write buffer"), w960) -> (w959:string)
        "concatenated string" <- w959
        n474 = VISA Write(VISA resource name=w963, write buffer=w959, error in (no error)=w962) -> (VISA resource name out=w958:refnum<visa-resource-name>, error out=w956:errorcluster)  [unwired: 1 out]
        n475 = VISA Write(VISA resource name=w958, write buffer="VOLTage:DC:AVERage:COUNt?", error in (no error)=w956) -> (VISA resource name out=w951:refnum<visa-resource-name>, error out=w955:errorcluster)  [unwired: 1 out]
        n476 = VISA Read(VISA resource name=w951, byte count=u32 100, error in (no error)=w955) -> (read buffer=w949:string, error out=w954:errorcluster)  [unwired: 2 out]
        n477 = Decimal String To Number(string=w949) -> (number=w948:i32)  [unwired: 2 in, 1 out]
        n478 = Equal?(x="Keithley (IV conv) averaging", y=w948) -> (x = y?=→"Confirm":bool)
      }
      event "Max Field (T)": Value Change {
        n479 = event-data() -> ()  [unwired: 1 in, 6 out]
        n480 = Divide(x="Max Field (T)", y="dB (T)") -> (x/y=w966:dbl)
        n481 = for {
          N: w966 -> [_]
          tunnel: "dB (T)" -> [w976]
          tunnel: [w973] -> w965 mode=indexing
          tunnel: "Min Field (T)" -> [w974]
          tunnel: [0.0] -> _ mode=indexing
          i -> [w977]
          n482 = Multiply(x=w977, y=w976) -> (x*y=w975:dbl)
          n483 = Add(x=w975, y=w974) -> (x+y=w973:dbl)
        }
        "B array" <- w965
      }
      event "Sweep Rate (T/min)": Value Change {
        n484 = event-data() -> ("NewVal"=w983:dbl)  [unwired: 1 in, 5 out]
        n485 = local read "Magnet"() -> (w978:bool)
        n486 = case shown="False" w978 {
          tunnel: w983 -> [_ w990]
          tunnel: w982 -> [w984 w986]
          tunnel: [w984 w985] -> w979
          frame False {
          }
          frame True {
            n487 = Number To Fractional String(number=w990, precision (6)=i16 3) -> (F-format string=w988:string)  [unwired: 2 in]
            n488 = Concatenate Strings("T" ("format string"), w988) -> (w987:string)
            n489 = call "GPIB - BusCommand.vi"("Command"=w987, "Address"=w986) -> ("Address(thru)"=w985:T6)  [unwired: 1 out]
          }
        }
      }
      event "Field To Zero": Value Change {
        n490 = event-data() -> ()  [unwired: 1 in, 6 out]
        n491 = Two Button Dialog(message="Do you want to switch off the field?", 1:"No" ("F button name (\"Cancel\")"), 2:"Yes" ("T button name (\"OK\")")) -> (T button?=w999:bool)
        n492 = case shown="True" w999 {
          tunnel: w994 -> [_ w1004]
          tunnel: w993 -> [w1000 w1002]
          tunnel: [w1000 w1001] -> w992
          frame False {
          }
          frame True {
            n493 = local read "Magnet"() -> (w1003:bool)
            n494 = case shown="False" w1003 {
              tunnel: w1004 -> [_ w1056]
              tunnel: w1002 -> [w1007 w1053]
              tunnel: [w1006 w1053] -> w1001
              frame False {
                n495 = local read "Lock_in_Amplifier"() -> (w1005:refnum<visa-resource-name>)
                n496 = stacked-sequence {
                  seq-local: [w1010 _] -> [_ w1022]
                  seq-local: [w1008 _] -> [_ w1019]
                  tunnel: w1007 -> [w1012 _]
                  tunnel: [_ w1025] -> w1006
                  tunnel: w1005 -> [w1009 w1020]
                  frame #0 {
                    n497 = VISA Write(VISA resource name=w1009, write buffer="AUXV?1", error in (no error)=w1012) -> (VISA resource name out=w1016:refnum<visa-resource-name>, error out=w1011:errorcluster)  [unwired: 1 out]
                    n498 = VISA Read(VISA resource name=w1016, byte count=u32 1000, error in (no error)=w1011) -> (read buffer=w1013:string, error out=w1010:errorcluster)  [unwired: 2 out]
                    n499 = Fract/Exp String To Number(string=w1013) -> (number=w1008:dbl)  [unwired: 3 in, 1 out]
                  }
                  frame #1 {
                    w1028 = 0.001 ("Voltage Step (V)")
                    n500 = local read "Sweep Rate (T/min)"() -> (w1027:dbl)
                    n501 = local read "V/I (Ohm)"() -> (w1024:dbl)
                    n502 = local read "B/V (T/V)"() -> (w1018:dbl)
                    n503 = xnode "Sweep Delay"("SweepRate"=w1027, "Resolution"=w1028, "BpV"=w1018) -> ("Result"=w1026:dbl)  [unwired: 1 in, 1 out]
                    n504 = call "Universal_Ramping.vi"("milliseconds to wait"=w1026, "Initial Voltage (V)"=w1019, "error in (no error)"=w1022, "Voltage Step (V)"=w1028, "Final Voltage (V)"=0.0, "VISA resource name"=w1020) -> ("error out"=w1025:errorcluster, "Actual Voltage (V)"=w1017:dbl)  [unwired: 3 in, 1 out]
                    n505 = local write "Actual Voltage (V)"(w1017) -> ()
                    n506 = xnode "AUXtoB"("BpV"=w1018, "Rm"=w1024, "Aux"=w1017) -> ("Result"=w1023:dbl)  [unwired: 1 in, 1 out]
                    n507 = local write "Actual B Field (T)"(w1023) -> ()
                  }
                }
              }
              frame True {
                n508 = local read "Sweep Rate (T/min)"() -> (w1055:dbl)
                n509 = call "ips_switchHeaterOff.vi"("Instrument address"=w1056, "Rate"=w1055) -> ("B"=w1054:dbl)
                n510 = local write "Actual Field (T)"(w1054) -> ()
              }
            }
          }
        }
      }
      event "Go to Set": Value Change {
        n511 = event-data() -> ()  [unwired: 1 in, 6 out]
        n512 = local read "V/I (Ohm)"() -> (w1063:dbl)
        n513 = local read "B/V (T/V)"() -> (w1062:dbl)
        n514 = local read "Lock_in_Amplifier"() -> (w1059:refnum<visa-resource-name>)
        n515 = local read "Sweep Rate (T/min)"() -> (w1061:dbl)
        n516 = local read "Magnet"() -> (w1064:bool)
        n517 = call "Ramp_Field.vi"("Set Field (T) in"="Set Field (T)", "Sweep Rate (T/min)"=w1061, "V/I (Ohm)"=w1063, "error in (no error)"=w1065, "Magnet"=w1064, "B/V (T/V)"=w1062, "VISA Refnum in"=w1059) -> ("error out"=w1067:errorcluster, "Actual Voltage (V)"=w1057:dbl, "Set Field (T) out"=w1060:dbl)  [unwired: 2 in]
        n518 = local write "Actual B Field (T)"(w1060) -> ()
        n519 = local write "Actual Voltage (V)"(w1057) -> ()
      }
      event "Measure /Pause": Value Change {
        n520 = event-data() -> ("NewVal"=w1069:bool)  [unwired: 1 in, 5 out]
        n521 = local write "Measuring"(w1069) -> ()
      }
      event "Stop": Value Change {
        n522 = event-data() -> ()  [unwired: 1 in, 6 out]
        n523 = local read "Measuring"() -> (w1077:bool)
        n524 = case shown="True" w1077 {
          tunnel: w1076 -> [w1078 w1081]
          tunnel: [w1078 w1082] -> w1075
          frame False {
          }
          frame True {
            w1089 = FALSE ("Measuring")
            n525 = local read "SaveSweep"() -> (w1090:bool)
            n526 = local write "Measuring"(w1089) -> ()
            n527 = local write "Measure /Pause"(w1089) -> ()
            n528 = local read "Lock_in_Amplifier"() -> (w1083:refnum<visa-resource-name>)
            n529 = case shown="True" w1090 {
              frame False {
              }
              frame True {
                w1096 = 1 ("index (row)")
                w1097 = 0 ("index (row)")
                n530 = local read "Measurement File_average"() -> (w1109:path)
                n531 = local read "Averaged P(B)"() -> (w1098:dbl[][])
                n532 = local read "Averaged dt"() -> (w1100:dbl[][])
                n533 = local read "I(B) /Averaged/"() -> (w1108:cluster{"B array":dbl[], dbl[]}[])
                n534 = Index Array(array=w1100, index (row)=w1097) -> (element=w1099:dbl[])  [unwired: 1 in]
                n535 = Index Array(array=w1100, index (row)=w1096) -> (element=w1092:dbl[])  [unwired: 1 in]
                n536 = Index Array(array=w1108, index=1) -> (element=w1104:cluster{"B array":dbl[], dbl[]})
                n537 = Index Array(array=w1108, index=0) -> (element=w1105:cluster{"B array":dbl[], dbl[]})
                n538 = Unbundle(w1104) -> ("B array"=w1094:dbl[], w1093:dbl[])
                n539 = Unbundle(w1105) -> ("B array"=w1103:dbl[], w1102:dbl[])
                n540 = Index Array(array=w1098, index (row)=w1097) -> (element=w1095:dbl[])  [unwired: 1 in]
                n541 = Index Array(array=w1098, index (row)=w1096) -> (element=w1091:dbl[])  [unwired: 1 in]
                n542 = Build Array(w1103, w1102, w1099, w1095, w1094, w1093, w1092, w1091) -> (w1101:dbl[][])
                n543 = call-poly <vilib>:"Write Delimited Spreadsheet.vi"("file path (dialog if empty)"=w1109, "format (%.3f)"="%.5g", "2D data"=w1101, "append to file? (F)"=TRUE ("transpose? (F)"), "transpose? (F)"=TRUE ("append to file? (F)")) -> ()  [unwired: 9 in, 2 out]
              }
            }
            n544 = local read "V/I (Ohm)"() -> (w1087:dbl)
            n545 = local read "Sweep Rate (T/min)"() -> (w1086:dbl)
            n546 = local read "Set Field (T)"() -> (w1088:dbl)
            n547 = local read "B/V (T/V)"() -> (w1084:dbl)
            n548 = local read "Magnet"() -> (w1085:bool)
            n549 = call "Ramp_Field.vi"("Set Field (T) in"=w1088, "Sweep Rate (T/min)"=w1086, "V/I (Ohm)"=w1087, "error in (no error)"=w1081, "Magnet"=w1085, "B/V (T/V)"=w1084, "VISA Refnum in"=w1083) -> ("error out"=w1082:errorcluster, "Actual Voltage (V)"=w1079:dbl, "Set Field (T) out"=w1080:dbl)  [unwired: 2 in]
            n550 = local write "Actual B Field (T)"(w1080) -> ()
            n551 = local write "Actual Voltage (V)"(w1079) -> ()
          }
        }
      }
      event "Sweep": Value Change {
        n552 = event-data() -> ("NewVal"=w1116:bool)  [unwired: 1 in, 5 out]
        n553 = case shown="True" w1116 {
          frame False {
          }
          frame True {
            n554 = local read "Measurement File"() -> (w1117:path)
            n555 = Two Button Dialog(message="Do you want to create additional files for the sweeping measurements?" ("string"), 1:"No" ("F button name (\"Cancel\")"), 2:"Yes" ("T button name (\"OK\")")) -> (T button?=w1119:bool)
            n556 = case shown="True" w1119 {
              tunnel: w1117 -> [_ w1124]
              frame False {
                n557 = local write "SaveSweep"(FALSE ("SaveSweep")) -> ()
              }
              frame True {
                n558 = call "Create_sweep_files.vi"("Measurement File"=w1124) -> ("Path 3"=→"Measurement File_dn":path, "Path 2"=→"Measurement File_up":path, "Path"=→"Measurement File_average":path)  [unwired: 8 in]
                "SaveSweep" <- TRUE
              }
            }
          }
        }
      }
      event "Measure Noise": Value Change {
        n559 = event-data() -> ("NewVal"=w1131:bool)  [unwired: 1 in, 5 out]
        n560 = case shown="True" w1131 {
          frame False {
          }
          frame True {
            n561 = local read "Gain (V/A)"() -> (w1136:dbl)
            n562 = call "Noise_measurement.vi"("Gain (V/A)"=w1136, "Cycles"="Cycles", "Lower Cut-Off"="Cut-Off Frequency", "minimum value"="minimum value", "Filter On"="Filter On", "maximum value"="maximum value", "physical channels"="physical channels", "rate"="Rate", "samples per channel"="Samples per channel") -> ("Current (pA) Filtered"=→"Current (pA) Filtered":waveform(dbl), "PSD (pA/Hz^1/2) Peaks Removed"=→"PSD (pA/Hz^1/2) Peaks Removed":cluster{"f0":dbl, "df":dbl, "magnitude":dbl[]}, "Current (pA)"=→"Current (pA)":dbl[], "PSD (pA/Hz^1/2)"=→"PSD (pA/Hz^1/2)":cluster{"f0":dbl, "df":dbl, "magnitude":dbl[]})  [unwired: 3 in]
          }
        }
      }
      event "Calibrate": Value Change {
        n563 = event-data() -> ()  [unwired: 1 in, 6 out]
        n564 = case shown="True" "Calibrate" {
          frame False {
          }
          frame True {
            w1151 = dbl[] []
            n565 = while {
              shift-right: [w1184] -> w1149
              shift-left: dbl[][] [] -> [w1183]
              shift-right: [w1167] -> _
              shift-left: w1151 -> [w1179]
              shift-right: [w1176] -> _
              shift-left: w1151 -> [w1178]
              shift-right: [w1166] -> _
              shift-left: w1151 -> [w1177]
              shift-right: [w1158] -> _
              shift-left: 0.0 ("Set Field out") -> [w1157]
              stop <- w1180 stop-if-true
              n566 = call "Calibtarion.vi"("Dwell Time (ms)"="Dwell Time (ms)", "V array in (V)"=w1179, "I array in (A)"=w1177, "Collected array in"=w1183, "B array in (T)"=w1178, "Set Field (T)"=w1157, "dB"="dB") -> ("Best Linear Fit"=w1168:dbl[], "appended array"=→"appended array":dbl[][], "slope"=→"B/V (T/V)":dbl, "V array out (V)"=w1167:dbl[], "Boolean"=w1182:bool, "I array out (A)"=w1166:dbl[], "intercept 2"=→"I0 (A)":dbl, "Collected array out"=w1184:dbl[][], "intercept"=→"B0 (T)":dbl, "B array Out"=w1176:dbl[], "slope 2"=→"V/I (Ohm)":dbl, "Best Linear Fit 2"=w1173:dbl[], "Set Field out"=w1158:dbl)
              n567 = Bundle("I array out (A)"=w1166, "V array out (V)"=w1167) -> (w1175:T11)  [unwired: 1 in]
              n568 = Bundle("I array out (A)"=w1166, "Best Linear Fit"=w1168) -> (w1169:T12)  [unwired: 1 in]
              n569 = Bundle("V array out (V)"=w1167, "B array Out"=w1176) -> (w1171:T13)  [unwired: 1 in]
              n570 = Bundle("V array out (V)"=w1167, "Best Linear Fit 2"=w1173) -> (w1172:T14)  [unwired: 1 in]
              n571 = Or(x=w1182, y="stop 2") -> (x .or. y?=w1180:bool)
              n572 = Build Array(w1175, w1169) -> (→"V_I":T15)
              n573 = Build Array(w1171, w1172) -> (→"B_V":T16)
            }
            n574 = flat-sequence {
              tunnel: w1149 -> [w1155]
              frame #0 {
                n575 = Two Button Dialog(message="Do you want to save calibration file?") -> (T button?=w1154:bool)  [unwired: 2 in]
                n576 = case shown="True" w1154 {
                  tunnel: w1155 -> [_ w1156]
                  frame False {
                  }
                  frame True {
                    n577 = call-poly <vilib>:"Write Delimited Spreadsheet.vi"("2D data"=w1156) -> ()  [unwired: 13 in, 2 out]
                  }
                }
              }
            }
          }
        }
      }
      event "New Measurement File": Value Change {
        n578 = event-data() -> ()  [unwired: 1 in, 6 out]
        n579 = local read "Sweep"() -> (w1186:bool)
        n580 = Open/Create/Replace File(prompt="Please select measurement file\n", operation (0:open)=T5."replace or create with confirmation") -> (refnum out=w1192:refnum<file>)  [unwired: 4 in, 2 out]
        n581 = local write "refnum out"(w1192) -> ()
        n582 = Refnum to Path(1:w1192) -> (0:w1187:path)
        n583 = case shown="True" w1186 {
          tunnel: w1187 -> [_ w1195]
          frame False {
          }
          frame True {
            n584 = Two Button Dialog(message="Do you want to create additional files for the sweeping measurements?" ("string"), 1:"No" ("F button name (\"Cancel\")"), 2:"Yes" ("T button name (\"OK\")")) -> (T button?=w1197:bool)
            n585 = case shown="True" w1197 {
              tunnel: w1195 -> [_ w1205]
              frame False {
                n586 = local write "SaveSweep"(FALSE ("SaveSweep")) -> ()
              }
              frame True {
                n587 = call "Create_sweep_files.vi"("Measurement File"=w1205) -> ("Path 3"=w1202:path, "Path 2"=w1203:path, "Path"=w1204:path)  [unwired: 8 in]
                n588 = local write "Measurement File_dn"(w1202) -> ()
                n589 = local write "Measurement File_average"(w1204) -> ()
                n590 = local write "Measurement File_up"(w1203) -> ()
                n591 = local write "SaveSweep"(TRUE) -> ()
              }
            }
          }
        }
        n592 = local write "Measurement File"(w1187) -> ()
        n593 = local write "Offset?"(FALSE ("Offset?")) -> ()
        n594 = local write "First?"(TRUE ("First?")) -> ()
      }
      event "Heater On/Off": Value Change {
        n595 = event-data() -> ()  [unwired: 1 in, 6 out]
        n596 = case shown="False" "Heater On/Off" {
          tunnel: w1210 -> [w1215 w1221]
          tunnel: w1209 -> [w1213 w1222]
          tunnel: [w1212 w1220] -> w1208
          frame False {
            n597 = VISA Write(VISA resource name=w1215, write buffer="RANGE,1,0", error in (no error)=w1213) -> (error out=w1212:errorcluster)  [unwired: 2 out]
          }
          frame True {
            n598 = Number To Decimal String(number="Heater Range") -> (decimal integer string=w1218:string)  [unwired: 1 in]
            n599 = Concatenate Strings("RANGE,1," ("write buffer"), w1218) -> (w1216:string)
            n600 = VISA Write(VISA resource name=w1221, write buffer=w1216, error in (no error)=w1222) -> (error out=w1220:errorcluster)  [unwired: 2 out]
          }
        }
      }
      event "Set temperature (K)": Value Change {
        n601 = event-data() -> ()  [unwired: 1 in, 6 out]
        n602 = local read "Set temperature (K)"() -> (w1228:dbl)
        n603 = Number To Fractional String(number=w1228, precision (6)=i16 3) -> (F-format string=w1231:string)  [unwired: 2 in]
        n604 = Concatenate Strings("SETP 1," ("write buffer"), w1231) -> (w1229:string)
        n605 = VISA Write(VISA resource name=w1225, write buffer=w1229, error in (no error)=w1227) -> (error out=w1226:errorcluster)  [unwired: 2 out]
      }
      event "Temp Ramping Rate (K/min)": Value Change {
        n606 = event-data() -> ()  [unwired: 1 in, 6 out]
        n607 = local read "Temp Ramping Rate (K/min)"() -> (w1235:dbl)
        n608 = Number To Fractional String(number=w1235, precision (6)=i16 1) -> (F-format string=w1241:string)  [unwired: 2 in]
        n609 = Concatenate Strings("RAMP 1,1," ("string"), w1241) -> (w1240:string)
        n610 = VISA Write(VISA resource name=w1238, write buffer=w1240, error in (no error)=w1237) -> (error out=w1236:errorcluster)  [unwired: 2 out]
      }
      event "Heater Range": Value Change {
        n611 = event-data() -> ()  [unwired: 1 in, 6 out]
        n612 = local read "Heater On/Off"() -> (w1247:bool)
        n613 = case shown="True" w1247 {
          tunnel: w1246 -> [w1248 w1253]
          tunnel: [w1248 w1252] -> w1245
          tunnel: w1243 -> [_ w1251]
          frame False {
          }
          frame True {
            n614 = local read "Heater Range"() -> (w1249:enum16{"Off", "Low", "Medium", "High"})
            n615 = Number To Decimal String(number=w1249) -> (decimal integer string=w1255:string)  [unwired: 1 in]
            n616 = Concatenate Strings("RANGE,1," ("write buffer"), w1255) -> (w1254:string)
            n617 = VISA Write(VISA resource name=w1251, write buffer=w1254, error in (no error)=w1253) -> (error out=w1252:errorcluster)  [unwired: 2 out]
          }
        }
      }
    }
    n618 = Reciprocal(x="Sampling rate (Hz)") -> (1/x=w890:dbl)
    n619 = Multiply(x=w890, y=1000.0) -> (x*y=w888:dbl)
    n620 = Wait Until Next ms Multiple(millisecond multiple=w888) -> ()  [unwired: 1 out]
  }
  n621 = local read "Max Field (T)"() -> (w67:dbl)
  n622 = local read "Min Field (T)"() -> (w69:dbl)
  n623 = local read "dB (T)"() -> (w68:dbl)
  n624 = Divide(x=w67, y=w68) -> (x/y=w70:dbl)
  n625 = for {
    N: w70 -> [_]
    tunnel: w68 -> [w1260]
    tunnel: [w1257] -> w30 mode=indexing
    tunnel: w69 -> [w1258]
    tunnel: [0.0] -> _ mode=indexing
    i -> [w1261]
    n626 = Multiply(x=w1261, y=w1260) -> (x*y=w1259:dbl)
    n627 = Add(x=w1259, y=w1258) -> (x+y=w1257:dbl)
  }
  n628 = Multiply(x=w30, y=0.0) -> (x*y=w27:dbl[])
  n629 = Array Size(array=w27) -> (size(s)=w26:i32)
  n630 = Decrement(x=w26) -> (x-1=w25:i32)
  n631 = local write "B array"(w30) -> ()
  n632 = Array Subset(array=w27, length=w25) -> (w24:dbl[])  [unwired: 1 in]
  n633 = Build Array(w27, w27) -> (w28:dbl[][])
  n634 = local write "Averaged I(B)"(w28) -> ()
  n635 = Build Array(w24, w24) -> (w23:dbl[][])
  n636 = local write "Averaged P(B)"(w23) -> ()
  n637 = local write "Averaged dt"(w23) -> ()
  n638 = local read "Lake Shore"() -> (w80:refnum<visa-resource-name>)
  n639 = local read "IV converter"() -> (w96:refnum<visa-resource-name>)
  n640 = local read "Magnetic Field"() -> (w95:refnum<visa-resource-name>)
  n641 = VISA Close(VISA resource name=w96, error in (no error)=w98) -> (error out=w99:errorcluster)
  n642 = VISA Close(VISA resource name=w95, error in (no error)=w99) -> (error out=w97:errorcluster)
  n643 = Release Queue(queue=w103, error in (no error)=w97) -> (error out=w93:errorcluster)  [unwired: 1 in, 2 out]
  n644 = Merge Errors(w93, w92) -> (w94:errorcluster)
  n645 = VISA Close(VISA resource name=w80, error in (no error)=w94) -> (error out=w91:errorcluster)
  n646 = local read "refnum out"() -> (w89:refnum<file>)
  n647 = Close File(refnum=w89, error in=w91) -> (error out=w90:errorcluster)  [unwired: 1 out]
  n648 = call <vilib>:"Simple Error Handler.vi"("error in (no error)"=w90) -> ()  [unwired: 4 in, 5 out]
  "i" <- w60
  "j" <- w60
